vi "Diagnostics.Main.CmdResp.Engine.vi"(8 "error in (no error)":errorcluster, 11 "State Variables":T1={"Comm"=refnum, "Parameters"={"Properties"={"Name"="", "CAN"={"Interface"="", "Baud Rate"=0, "Diagnostic Protocol"=enum."GMLAN", "Transport Protocol"=enum."ISO TP - Normal Mode", "Transmit ID"=0, "Receive ID"=0, "Transmit Extension"=2, "Receive Extension"=1, "Receive UUDT ID"=0, "Enable Stream"=TRUE, "VW TP Channel ID"=0, "Fill Frame"=FALSE, "Fill Byte"=255, "Termination"=FALSE, "LIN Cluster"="ADCS_LIN_database", "NAD"=1, "IO Mode"=0, "Max DLC"=8, "FD Baud Rate"=0, "Security"={"Type"=enum."None", "Source DLL Path"=path "", "Target DLL Path"=path "", "Security Level"=0, "Master Key"=""}, "Timeout"=0}, "986x"={"Enable"=FALSE, "RIO Device"="", "Bitfile"=path ""}, "Reads"=[], "Frames Lookup"=variant(enum16{"GMLAN", "KWP-2000", "UDS"} enum."GMLAN"), "Writes"=[], "DPIDs"=[], "DPID Lookup"=variant(u32 0), "DTC"={"Descriptor"={"DTC Byte Length"=2, "Status Byte Length"=1, "Add Data Byte Length"=1, "Byte Order"=enum."Motorola"}, "Value.Code"=[], "Value.String"=[], "Value.J2012String"=[], "Status.Code"=[], "Status.String"=[]}, "Created DTCs"=0, "Polls"=[], "Service Channels Status Lookup"=variant, "Trigger Lookup"=variant}}, "ADCS Connection"={"Diag CAN Handle"=0, "Transport Protocol"=enum."ISO TP - Normal Mode", "Receive Address Extension"=0, "Transmit Address Extension"=0, "Receive CAN Id"=0, "Transmit CAN Id"=0, "Log Frames ?"=FALSE, "My TP Address"=0, "Other TP Address"=0, "T1"=0, "T2"=0, "T3"=0, "T4"=0, "Tx SN"=0, "Block Size"=0, "Rx SN"=0, "VW TP Initialized?"=FALSE, "Tx block no"=0, "baud rate"=0, "Interface"="", "Channel Diag CAN Handle"=0, "UDP Connection ID"=refnum, "TCP Connection ID"=refnum, "Target IP Addr"=0, "Source Address"=0, "Target Address"=0, "Send Header NACK?"=FALSE, "DLL Handle"=0, "NAD"=0, "Time Stamp read first"=0.0, "Time Stamp read last"=0.0, "Time Stamp write first"=0.0, "Time Stamp write last"=0.0, "Time Stamp write"=0.0, "Time Stamp read"=0.0, " I/O Mode"=0, "FD Baudrate"=0, "TX_DL"=8, "RX_DL"=8, "DoIP Protocol Version"=1, " Selected I/O Mode"=0, "TesterPresent Counter"=0, "TesterPresent Limit"=0, "TesterPresent Tick[ms]"=10, "TesterPresent RequireResponse?"=FALSE, "TesterPresent Stored Ref?"=FALSE, "TesterPresent Message"=[], "TesterPresent Task Handle"=0, "TesterPresent Semaphore"=refnum, "Response Plausibility Check"=1, "Default Version?"=TRUE, "Diagostic Globals"={"Timeout FC (Bs)"=250, "Timeout CF (Cr)"=250, "Timeout Diag Command"=1000, "Receive Block Size (BS)"=0, "Wait Time CF (STmin)"=5, "Max Waits (N_WFTmax)"=10, "Waits to Send (N_WAIT)"=0, "Time between Waits (TW)"=25, "Fill CAN Frames?"=TRUE, "Fill Byte"=255, "Invalid Response as Error?"=FALSE, "Max RspPending Count"=5, "VWTP Command Timeout"=50, "Transport Protocol"=enum."Diagnostics on IP", "Diag CAN Handle"=0, "DLL Handle"=0, "Timeout RspPending"=1000}, "Session-based Properties?"=FALSE}, "XNET References"={"Database"="", "GMLAN DPID Session"="", "Cluster"=""}, "XNETEngine (GMLAN)"=refnum, "Process"=refnum, "Reads"=refnum, "Writes"=refnum, "Cmds"=refnum, "DTCs"=refnum, "DTC Count"=refnum, "Status"=refnum, "Triggers"=refnum, "CANConnected"=refnum, "LocalStop"=refnum, "LocalCommStatus"=refnum, "Service Channels Status"=refnum, "Settings"=refnum} {"ADCS Connection"."Diagostic Globals"."Fill Byte" format="%x"; "ADCS Connection"."TesterPresent Message" format="%.0x"; "ADCS Connection"."Selected I/O Mode" items=["CAN", "CAN FD", "CAN FD+BRS", "ECU Determined"]; "ADCS Connection"."DoIP Protocol Version" items=["2010"=1, "2012"=2]; "ADCS Connection"."RX_DL" items=["8"=8, "12"=12, "16"=16, "20"=20, "24"=24, "32"=32, "48"=48, "64"=64]; "ADCS Connection"."TX_DL" items=["8"=8, "12"=12, "16"=16, "20"=20, "24"=24, "32"=32, "48"=48, "64"=64]; "ADCS Connection"."I/O Mode" items=["CAN", "CAN FD", "CAN FD+BRS", "Not yet determined"]; "Parameters"."Properties"."Writes"."Signals"."Byte Order" items=["Little Endian", "Big Endian"]; "Parameters"."Properties"."Writes"."Signals"."Data Type" items=["Signed", "Unsigned", "IEEE Float"]; "Parameters"."Properties"."CAN"."IO Mode" items=["CAN 2.0", "CAN FD", "CAN FD+BRS"]; "Parameters"."Properties"."CAN"."Fill Byte" format="%.0x"; "Parameters"."Properties"."CAN"."VW TP Channel ID" format="%.0x"; "Parameters"."Properties"."CAN"."Receive UUDT ID" format="%.0x"; "Parameters"."Properties"."CAN"."Receive Extension" format="%.0x"; "Parameters"."Properties"."CAN"."Transmit Extension" format="%.0x"; "Parameters"."Properties"."CAN"."Receive ID" format="%.0x"; "Parameters"."Properties"."CAN"."Transmit ID" format="%.0x"; "Parameters"."Properties"."Reads"."Signals"."Byte Order" items=["Little Endian", "Big Endian"]; "Parameters"."Properties"."Reads"."Signals"."Data Type" items=["Signed", "Unsigned", "IEEE Float"]}) -> (0 "error out":errorcluster)   [LabVIEW 2019, in "Diagnostics Addon Engine.lvlib"]
doc: "Async loop that handles the UDS commands sent either by the channel engine or the TCP engine"
uses:
  Diagnostics Addon Engine.lvlib
  <vilib>/NI VeriStand/Custom Device Tools/Custom Device Utility Library/Custom Device Utility Library.lvlib
  Shared/Types/DTC.Info.ctl
  Shared/Diagnostics Addon Shared.lvlib
  <vilib>/NI/AMC/AMC.lvlib
  GMLAN/GMLAN.lvlib
  GMLAN/_SubVIs/InitiateDiagnosticOperation_Parameter.ctl
  GMLAN/_SubVIs/InitiateDiagnosticOperation_SubFunctions.ctl
  GMLAN/_SubVIs/ReadDataByPacketIdentifier_SubFunctions.ctl
  <vilib>/Automotive Diagnostic Command Set/Diagnostic Transport.llb/Property ID.ctl
  <vilib>/addons/Automotive Diagnostic Command Set/NI_Automotive Diagnostic Command Set.lvlib
  Types/Frame.Data.ctl
  Shared/Types/Command.ReadDTCbyDTCNumber.ctl
  GMLAN/_SubVIs/ReadFailureRecordData_readFailureRecordParameters_failureRecordIdentifier.ctl
  Shared/Types/Command.IO.ctl
  Shared/Types/Type.ctl
  GMLAN/_SubVIs/TesterPresent_Parameter.ctl
  Shared/Types/Command.Communication.ctl
  Shared/Types/Command.Memory.ctl
  Shared/Types/Command.PassThru.Channel.ctl
  Shared/Types/Command.ReadDTC.ctl
  GMLAN/_SubVIs/DisableNormalCommunication_Parameter.ctl
  <vilib>/NI/NIVS Inline Async API/_VS Inline Async API/Process/Process.lvclass
  <vilib>/NI/NIVS Inline Async API/_Data Access Engine/Data Access Engine/Data Access Engine.lvclass
  <vilib>/NI/NIVS Inline Async API/_Data Access Engine/Data Access Engine/Methods/Write.Data.vi
  <vilib>/NI/NIVS Addon Network Comm/Engine/VeriStand Comm.lvclass
  Shared/Types/DTC.Descriptor.Override.ctl
  Shared/Types/Command.ClearDTC.ctl
  Shared/Types/Command.ControlDTC.ctl
  <vilib>/NI/NIVS Inline Async API/_Data Access Engine/Data Access Engine/Methods/Write.Data.Commit.vi
  Types/Polling.States.ctl
  Shared/Types/Signal.ctl
  Shared/Types/DPID.Rate.ctl
  Shared/Types/DPID.ctl
  Shared/Types/Protocol.ctl
  Shared/Types/CAN.Interface.ctl
  Shared/Types/CAN.ctl
  Shared/Types/SysDef.Compile.Properties.ctl
  Types/XNET.Refs.ctl
  Types/Diagnostics.State.ctl
  <vilib>/NI/Tools/Keyed Array/KeyedArray.ctl
  <vilib>/NI/Tools/Keyed Array/Tools_KeyedArray.lvlib
  <vilib>/NI/AMC/Message.ctl
  <vilib>/NI/AMC/Message Queue.ctl
  Shared/Types/Transport.ctl
  <vilib>/Automotive Diagnostic Command Set/Diagnostic Transport.llb/Transport Protocol Selector.ctl
  <vilib>/Automotive Diagnostic Command Set/Diagnostic Transport.llb/Diag Reference.ctl
  Shared/Types/Security.ctl
  Shared/Types/Frame.Compile.ctl
  Shared/Types/DTC.Settings.ctl
  Shared/Types/986x.ctl
  <vilib>/NI/NIVS Inline Async API/_Data Access Engine/Access Type Classes/ReadWrite/ReadWrite.lvclass
  Shared/Types/SysDef.Compile.ctl
  <vilib>/NI/NIVS Inline Async API/_Data Access Engine/Access Type Classes/Write/Write.lvclass
  <vilib>/NI/NIVS Inline Async API/_Data Access Engine/Data Access Engine/Types/Write.DVR.ctl
  <vilib>/NI/NIVS Inline Async API/_Data Access Engine/Access Type Classes/Read/Read.lvclass
  <vilib>/NI/NIVS Inline Async API/_Data Access Engine/Data Access Engine/Types/Read.DVR.ctl
  <vilib>/NI/NIVS Inline Async API/_Data Access Engine/Data Access Engine/Types/ReadWrite.DVR.ctl
  Shared/Types/DTC.Descriptor.ctl
  <vilib>/Automotive Diagnostic Command Set/Diagnostic Transport.llb/DoIP Protocol Version.ctl
  <vilib>/Automotive Diagnostic Command Set/Diagnostic Transport.llb/Diag Globals.ctl
  Shared/Types/Security.Type.ctl
  Shared/Types/Poll.Compiled.ctl
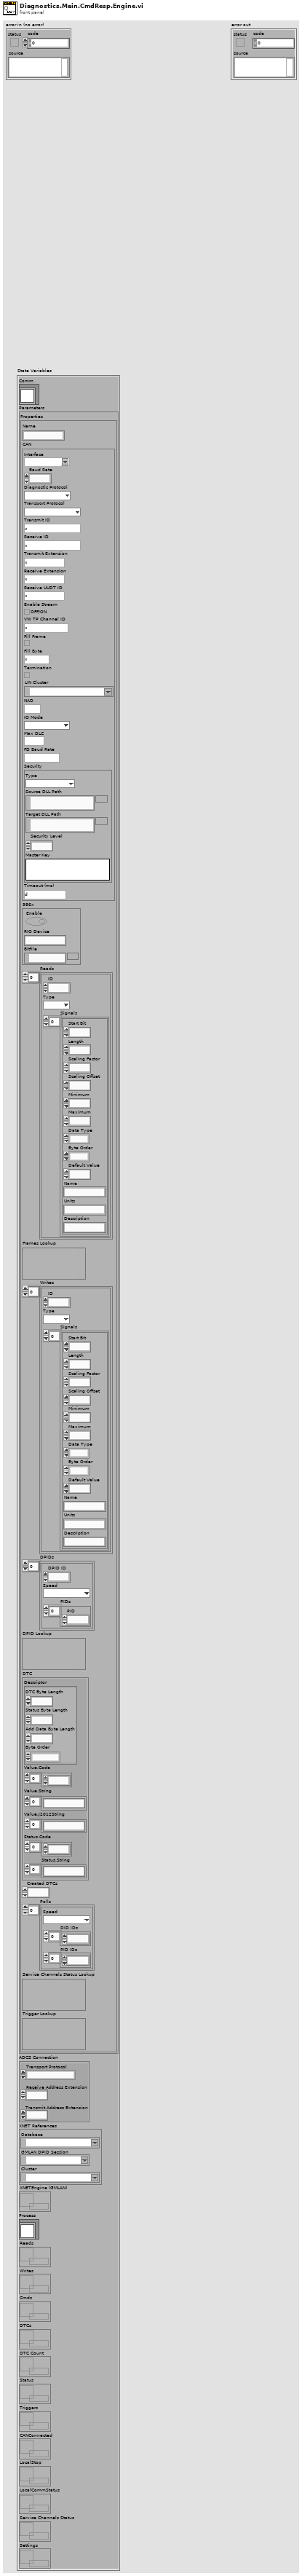
[diagram p1: front panel]
types:
  T1 = typedef "Diagnostics Addon Engine.lvlib/Diagnostics.State.ctl" = cluster{"Comm":refnum<class "VeriStand Comm.lvclass">, "Parameters":T2, "ADCS Connection":T19, "XNET References":T24, "XNETEngine (GMLAN)":T25, "Process":refnum<class "Process.lvclass">, "Reads":T26, "Writes":T27, "Cmds":T28, "DTCs":T26, "DTC Count":T26, "Status":T26, "Triggers":T28, "CANConnected":T26, "LocalStop":refnum<data-value>, "LocalCommStatus":refnum<data-value>, "Service Channels Status":T26, "Settings":T27}
  T2 = typedef "Diagnostics Addon Shared.lvlib/SysDef.Compile.ctl" = cluster{"Properties":T3}
  T3 = typedef "Diagnostics Addon Shared.lvlib/SysDef.Compile.Properties.ctl" = cluster{"Name":string, "CAN":T4, "986x":T10, "Reads":T11[], "Frames Lookup":variant, "Writes":T11[], "DPIDs":T14[], "DPID Lookup":variant, "DTC":T16, "Created DTCs":u32, "Polls":T18[], "Service Channels Status Lookup":variant, "Trigger Lookup":variant}
  T4 = typedef "Diagnostics Addon Shared.lvlib/CAN.ctl" = cluster{"Interface":T5, "Baud Rate":u64, "Diagnostic Protocol":T6, "Transport Protocol":T7, "Transmit ID":u32, "Receive ID":u32, "Transmit Extension":u8, "Receive Extension":u8, "Receive UUDT ID":u32, "Enable Stream":bool, "VW TP Channel ID":u32, "Fill Frame":bool, "Fill Byte":u8, "Termination":bool, "LIN Cluster":refnum<k21>, "NAD":u8, "IO Mode":u32, "Max DLC":u16, "FD Baud Rate":u64, "Security":T8, "Timeout":u32}
  T5 = typedef "Diagnostics Addon Shared.lvlib/CAN.Interface.ctl" = string
  T6 = typedef "Diagnostics Addon Shared.lvlib/Protocol.ctl" = enum16{"GMLAN", "KWP-2000", "UDS", "User-Defined"}
  T7 = typedef "Diagnostics Addon Shared.lvlib/Transport.ctl" = enum16{"ISO TP - Normal Mode", "ISO TP - Mixed Mode", "VW TP 2.0", "Diagnostics on IP", "ISO TP LIN"}
  T8 = typedef "Diagnostics Addon Shared.lvlib/Security.ctl" = cluster{"Type":T9, "Source DLL Path":path, "Target DLL Path":path, "Security Level":u8, "Master Key":string}
  T9 = typedef "Diagnostics Addon Shared.lvlib/Security.Type.ctl" = enum16{"None", "DLL", "MasterKey"}
  T10 = typedef "Diagnostics Addon Shared.lvlib/986x.ctl" = cluster{"Enable":bool, "RIO Device":string, "Bitfile":path}
  T11 = typedef "Diagnostics Addon Shared.lvlib/Frame.Compile.ctl" = cluster{"ID":u32, "Type":T12, "Signals":T13[]}
  T12 = typedef "Diagnostics Addon Shared.lvlib/Type.ctl" = enum16{"DID", "CDID", "PID", "CPID", "Read Memory", "Write Memory", "DTC Control", "IO Control", "Routine Start", "Routine Request", "Routine Stop", "User Defined", "Tester Present", "Clear DTCs", "Read DTCs", "Start DTCs", "DTC Change Count", "Unlock ECU", "Reset ECU", "Diagnostic Session Control", "Normal Communication Control", "Configure and Start DPIDs", "Stop DPIDs"}
  T13 = typedef "Diagnostics Addon Shared.lvlib/Signal.ctl" = cluster{"Start Bit":u32, "Length":u32, "Scaling Factor":dbl, "Scaling Offset":dbl, "Minimum":dbl, "Maximum":dbl, "Data Type":u32, "Byte Order":u32, "Default Value":dbl, "Name":string, "Units":string, "Description":string}
  T14 = typedef "Diagnostics Addon Shared.lvlib/DPID.ctl" = cluster{"DPID ID":u8, "Speed":T15, "PIDs":u16[]}
  T15 = typedef "Diagnostics Addon Shared.lvlib/DPID.Rate.ctl" = enum16{"Slow", "Medium", "Fast"}
  T16 = typedef "Diagnostics Addon Shared.lvlib/DTC.Settings.ctl" = cluster{"Descriptor":T17, "Value.Code":dbl[], "Value.String":string[], "Value.J2012String":string[], "Status.Code":dbl[], "Status.String":string[]}
  T17 = typedef "Diagnostics Addon Shared.lvlib/DTC.Descriptor.ctl" = cluster{"DTC Byte Length":i32, "Status Byte Length":i32, "Add Data Byte Length":i32, "Byte Order":enum16{"Motorola", "Intel"}}
  T18 = typedef "Diagnostics Addon Shared.lvlib/Poll.Compiled.ctl" = cluster{"Speed":T15, "DID IDs":u32[], "PID IDs":u32[]}
  T19 = typedef "NI_Automotive Diagnostic Command Set.lvlib/Diag Reference.ctl" = cluster{"Diag CAN Handle":u32, "Transport Protocol":T20, "Receive Address Extension":u8, "Transmit Address Extension":u8, "Receive CAN Id":u32, "Transmit CAN Id":u32, "Log Frames ?":bool, "My TP Address":u8, "Other TP Address":u8, "T1":u16, "T2":u16, "T3":u16, "T4":u16, "Tx SN":u8, "Block Size":u8, "Rx SN":u8, "VW TP Initialized?":bool, "Tx block no":u8, "baud rate":u64, "Interface":string, "Channel Diag CAN Handle":u32, "UDP Connection ID":refnum<k16>, "TCP Connection ID":refnum<k5>, "Target IP Addr":u32, "Source Address":u16, "Target Address":u16, "Send Header NACK?":bool, "DLL Handle":u32, "NAD":u8, "Time Stamp read first":dbl, "Time Stamp read last":dbl, "Time Stamp write first":dbl, "Time Stamp write last":dbl, "Time Stamp write":dbl, "Time Stamp read":dbl, " I/O Mode":u32, "FD Baudrate":u64, "TX_DL":u16, "RX_DL":u16, "DoIP Protocol Version":T21, " Selected I/O Mode":u32, "TesterPresent Counter":u32, "TesterPresent Limit":u32, "TesterPresent Tick[ms]":i32, "TesterPresent RequireResponse?":bool, "TesterPresent Stored Ref?":bool, "TesterPresent Message":u8[], "TesterPresent Task Handle":i32, "TesterPresent Semaphore":T22, "Response Plausibility Check":u32, "Default Version?":bool, "Diagostic Globals":T23, "Session-based Properties?":bool}
  T20 = typedef "NI_Automotive Diagnostic Command Set.lvlib/Transport Protocol Selector.ctl" = enum16{"ISO TP - Normal Mode", "ISO TP - Mixed Mode", "VW TP 2.0", "Diagnostics on IP", "ISO TP LIN"}
  T21 = typedef "NI_Automotive Diagnostic Command Set.lvlib/DoIP Protocol Version.ctl" = u8
  T22 = typedef "Semaphore RefNum" = refnum<k1>
  T23 = typedef "NI_Automotive Diagnostic Command Set.lvlib/Diag Globals.ctl" = cluster{"Timeout FC (Bs)":u32, "Timeout CF (Cr)":u32, "Timeout Diag Command":u32, "Receive Block Size (BS)":u8, "Wait Time CF (STmin)":u8, "Max Waits (N_WFTmax)":u8, "Waits to Send (N_WAIT)":i32, "Time between Waits (TW)":u32, "Fill CAN Frames?":bool, "Fill Byte":u32, "Invalid Response as Error?":bool, "Max RspPending Count":u32, "VWTP Command Timeout":u32, "Transport Protocol":T20, "Diag CAN Handle":u32, "DLL Handle":u32, "Timeout RspPending":u32}
  T24 = typedef "Diagnostics Addon Engine.lvlib/XNET.Refs.ctl" = cluster{"Database":refnum<k21>, "GMLAN DPID Session":refnum<k21>, "Cluster":refnum<k21>}
  T25 = typedef "AMC.lvlib/Message Queue.ctl" = refnum<queue>
  T26 = typedef "Data Access Engine.lvlib/Data Access Engine.lvclass/Write.DVR.ctl" = refnum<data-value>
  T27 = typedef "Data Access Engine.lvlib/Data Access Engine.lvclass/Read.DVR.ctl" = refnum<data-value>
  T28 = typedef "Data Access Engine.lvlib/Data Access Engine.lvclass/ReadWrite.DVR.ctl" = refnum<data-value>
  T29 = typedef "Diagnostics Addon Engine.lvlib/Polling.States.ctl" = cluster{"Enabled":bool[], "Last Generation":u32[], "Queued":bool[]}
  T30 = typedef "Diagnostics Addon Shared.lvlib/DTC.Info.ctl" = cluster{"Timestamp":dbl, "DTC":dbl, "Status":dbl, "Add Data":dbl}
  T31 = cluster{"Active DTCs":T30[], "status mask":u8, "PID IDs":u32[], "DID IDs":u32[], "Memory IDs":u32[], "TesterPresentEnabled?":bool, "Polling":T29}
  T32 = typedef "NI_Automotive Diagnostic Command Set.lvlib/Property ID.ctl" = enum16{"Timeout Diag Command", "Timeout FC (Bs)", "Timeout CF (Cr)", "Receive Block Size (BS)", "Wait Time CF (STmin)", "Max Wait Frames (N_WFTmax)", "Wait Frames to Send (N_WAIT)", "Time between Waits (T_W)", "Fill CAN Frames", "Fill Byte", "Invalid Response as Error", "Max RspPending Count", "VWTP Command Timeout", "STmin", "P2min", "Termination", "Timeout RspPending", "LIN Sleep", "Actual CAN IO Mode", "Response Plausibility Check", "Session-based Properties"}
  T33 = typedef "GMLAN.lvlib/ReadFailureRecordData_readFailureRecordParameters_failureRecordIdentifier.ctl" = cluster{"failureRecordNumber":u8, "DTC ID":u16, "DTCFailureType":u8}
  T34 = enum16{"open", "replace", "create", "open or create", "replace or create", "replace or create with confirmation"}
  T35 = typedef "Diagnostics Addon Shared.lvlib/Command.ReadDTCbyDTCNumber.ctl" = cluster{"DTC":u16, "FailTypeByte":u8}
  T36 = typedef "Diagnostics Addon Engine.lvlib/Frame.Data.ctl" = cluster{"ID":u32, "Raw Frame":u8[], "error out":errorcluster}
  T37 = typedef "GMLAN.lvlib/ReadDataByPacketIdentifier_SubFunctions.ctl" = enum8{"stopSending", "sendOneResponse", "scheduleAtSlowRate", "scheduleAtMediumRate", "scheduleAtFastRate"}
  T38 = typedef "GMLAN.lvlib/TesterPresent_Parameter.ctl" = enum8{"SpecificECU", "EntireNetwork"}
  T39 = typedef "GMLAN.lvlib/InitiateDiagnosticOperation_Parameter.ctl" = enum8{"SpecificECU", "EntireNetwork"}
  T40 = typedef "Diagnostics Addon Shared.lvlib/Command.Communication.ctl" = cluster{"Type":u8, "CommType":u8}
  T41 = typedef "GMLAN.lvlib/DisableNormalCommunication_Parameter.ctl" = enum8{"SpecificECU", "EntireNetwork"}
  T42 = typedef "Diagnostics Addon Shared.lvlib/Command.ReadDTC.ctl" = cluster{"Extension":u32, "Mask":u32, "Mode":u32, "Byte Lengths":T43}
  T43 = typedef "Diagnostics Addon Shared.lvlib/DTC.Descriptor.Override.ctl" = cluster{"Override":bool, "DTC":u32, "Status":u32, "Failure":u32}
  T44 = typedef "Diagnostics Addon Shared.lvlib/Command.ClearDTC.ctl" = cluster{"Group of DTC":u32, "Byte Lengths":T43}
  T45 = typedef "Diagnostics Addon Shared.lvlib/Command.PassThru.Channel.ctl" = cluster{"Service":u64, "Service Length":u8, "Data Length":u32, "Response Required":bool}
  T46 = cluster{"resp":u8[], "error code":u8, "error out":errorcluster}
  T47 = typedef "Diagnostics Addon Shared.lvlib/Command.ControlDTC.ctl" = cluster{"Group/Type":u32, "Byte Lengths (KWP only)":T43}
  T48 = typedef "Diagnostics Addon Shared.lvlib/Command.Memory.ctl" = cluster{"Address":u64, "Service Type":u32, "Address Length":u8, "Size Length":u8}
  T49 = typedef "Diagnostics Addon Shared.lvlib/Command.IO.ctl" = cluster{"ID":u16, "Mode":u8}
  T50 = typedef "NI VeriStand Addon Network Comm.lvlib/VeriStand Comm.lvclass/Response Information.ctl" = cluster{"response name":string, "responseQ":string}
  T51 = cluster{"Boolean array[0]":bool, "Boolean array[1]":bool, "Boolean array[2]":bool, "Boolean array[3]":bool, "Boolean array[4]":bool, "Boolean array[5]":bool, "Boolean array[6]":bool, "Boolean array[7]":bool}
  T52 = typedef "Diagnostics Addon Engine.lvlib/DPIDs.IDs.Sorted.ctl" = cluster{"Slow":u8[], "Medium":u8[], "Fast":u8[]}
  T53 = typedef "GMLAN.lvlib/InitiateDiagnosticOperation_SubFunctions.ctl" = u8
  T54 = typedef "Diagnostic Trouble Code.ctl" = cluster{"DTC":u32, "Status":u32, "Add Data":u32}
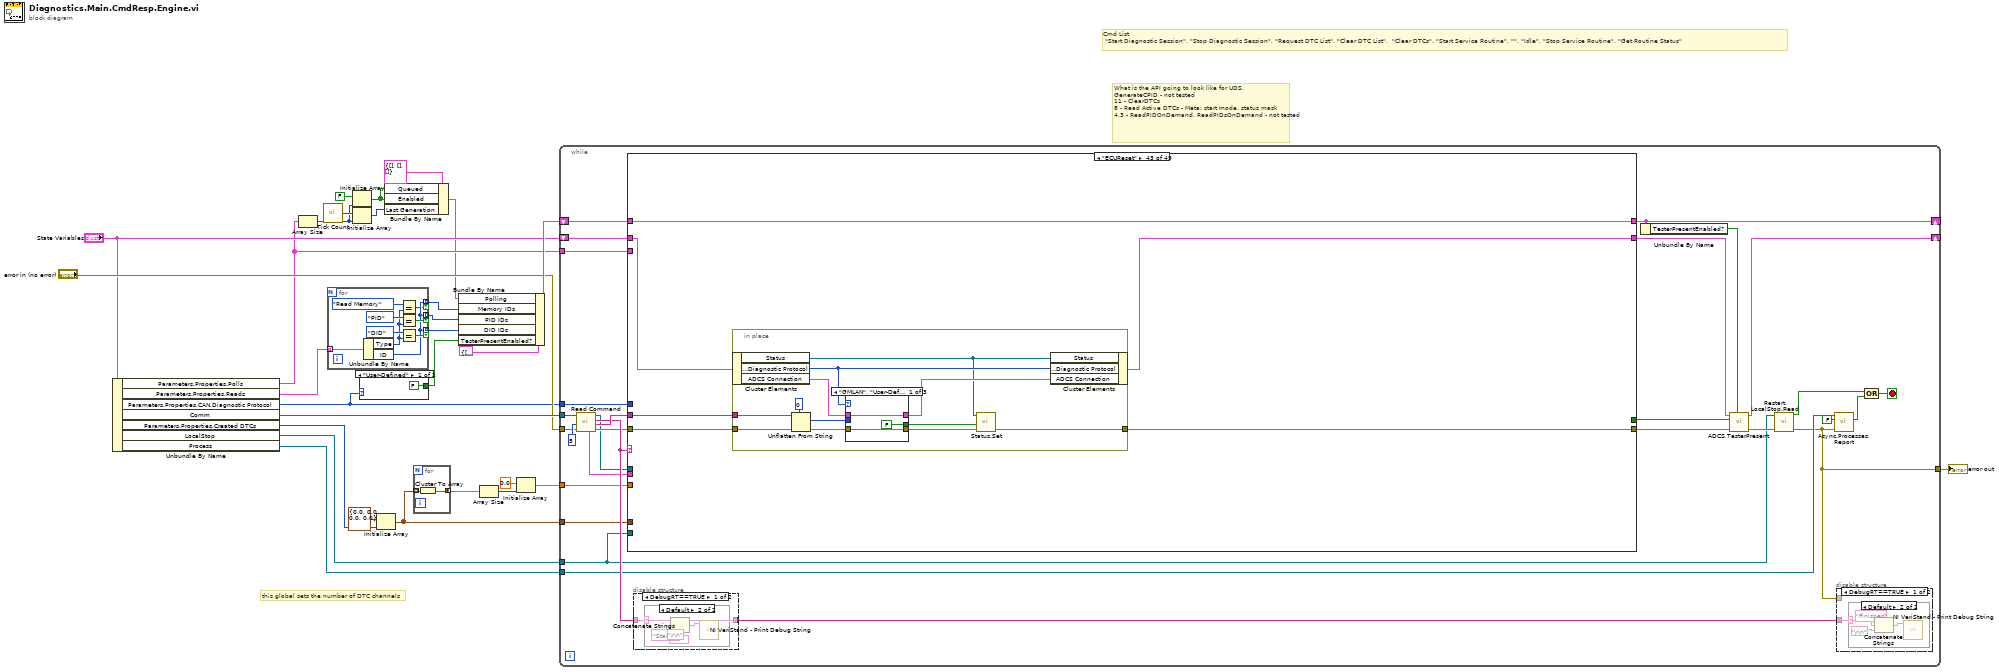
[diagram p0: block diagram]
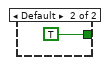
[diagram p2: hidden frame]
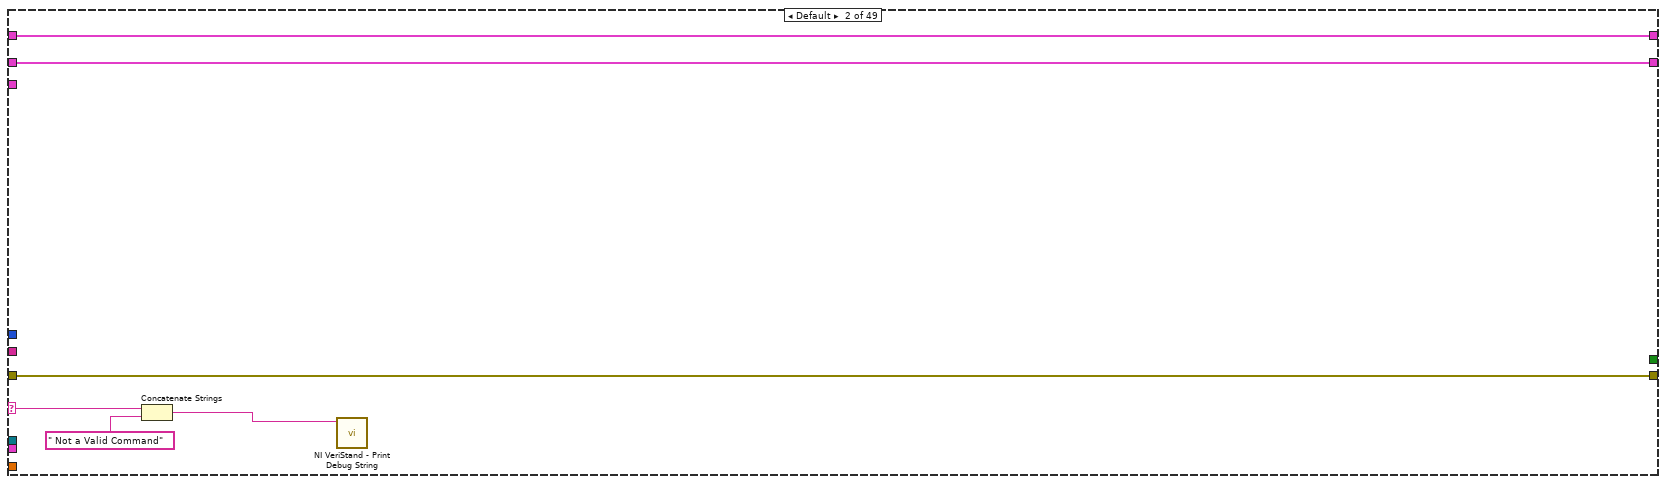
[diagram p8: hidden frame]
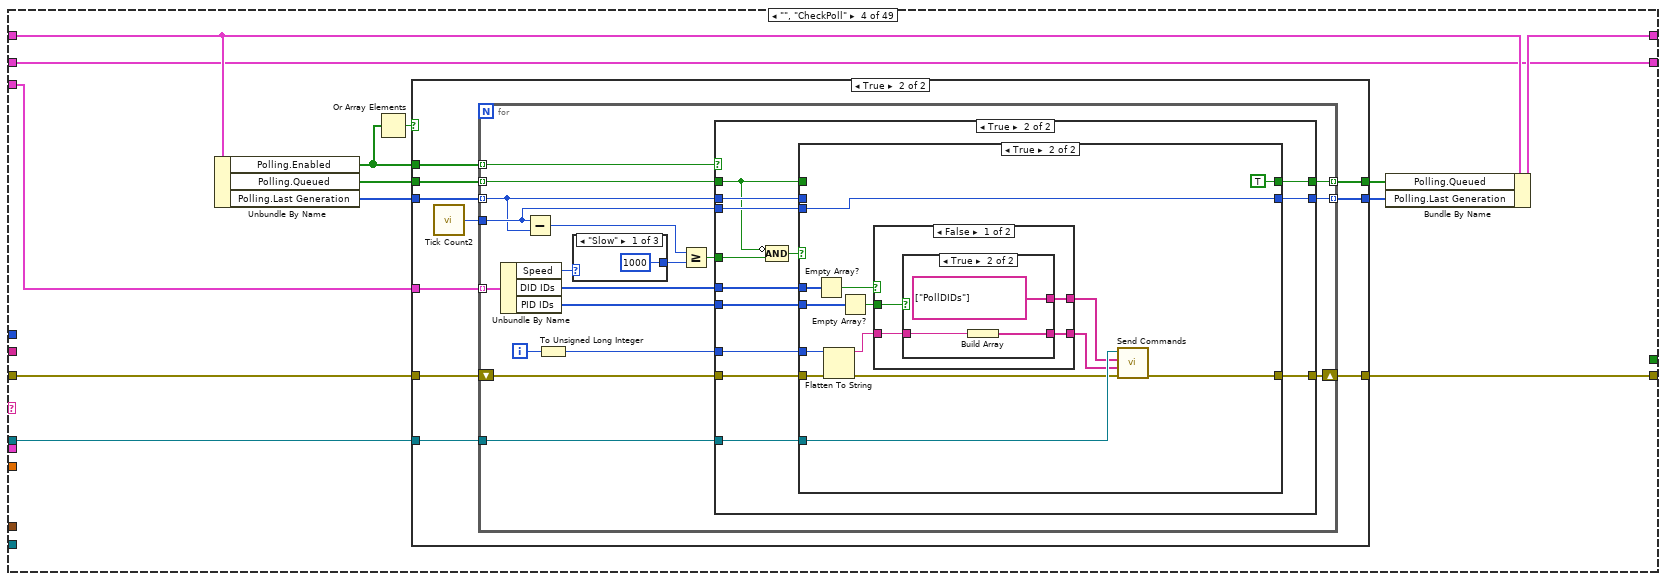
[diagram p10: hidden frame]
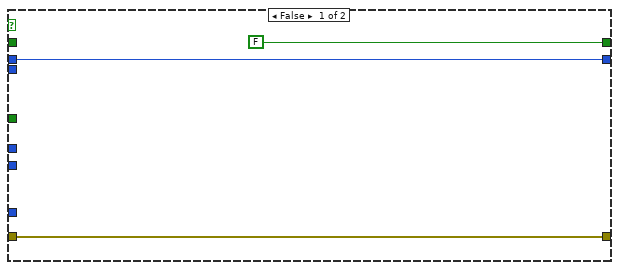
[diagram p12: hidden frame]
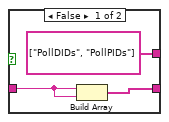
[diagram p14: hidden frame]
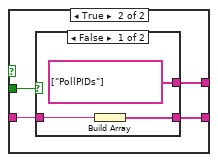
[diagram p15: hidden frame]
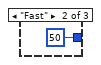
[diagram p17: hidden frame]
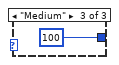
[diagram p18: hidden frame]
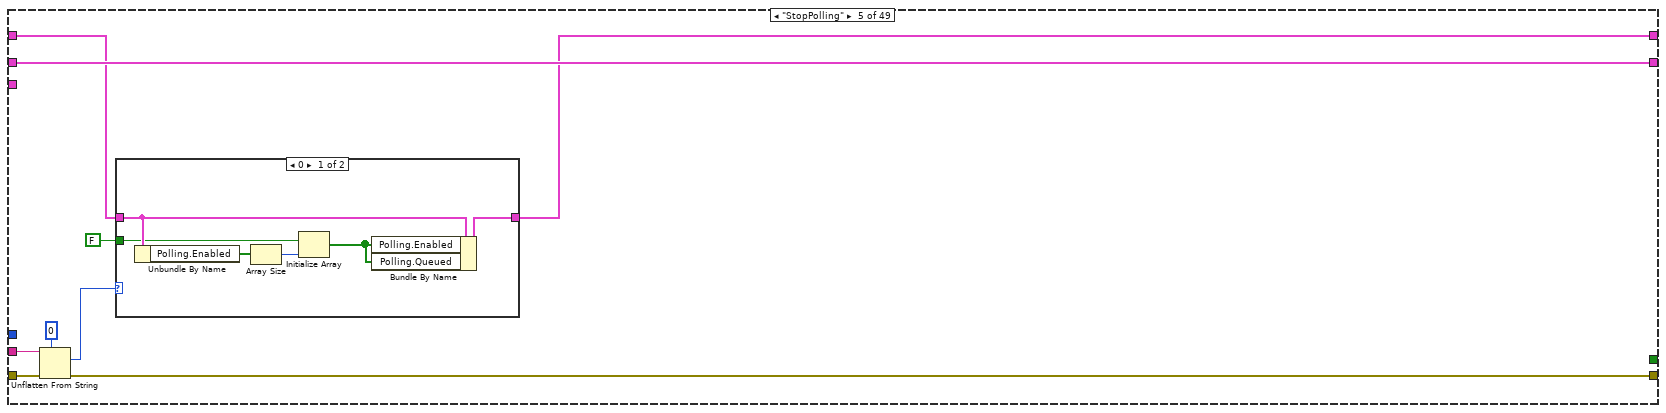
[diagram p19: hidden frame]
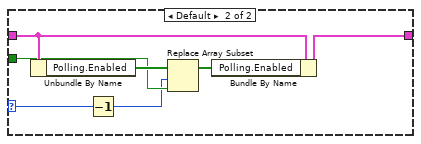
[diagram p20: hidden frame]
diagram:
  # "this global sets the number of DTC channels"
  # "What is the API going to look like for UDS.\nGenerateCPID - not tested\n11 - ClearDTCs\n8 - Read Active DTCs - Meta: start mode, status mask \n4,3 - ReadPIDOnDemand, ReadPIDsOnDemand - not tested"
  # "Cmd List\n \"Start Diagnostic Session\", \"Stop Diagnostic Session\", \"Request DTC List\", \"Clear DTC List\",  \"Clear DTCs\", \"Start Service Routine\", \"\", \"Idle\", \"Stop Service Routine\", \"Get Routine Status\""
  n1 = Unbundle By Name("State Variables") -> ("Parameters.Properties.Polls"=w5:T18[], "Parameters.Properties.Reads"=w26:T11[], "Parameters.Properties.CAN.Diagnostic Protocol"=w2:T6, "Comm"=w28:refnum<class "VeriStand Comm.lvclass">, "Parameters.Properties.Created DTCs"=w19:u32, "LocalStop"=w12:refnum<data-value>, "Process"=w18:refnum<class "Process.lvclass">)
  n2 = Array Size(array=w5) -> (size(s)=w6:i32)
  n3 = call "Tick Count"() -> ("Tick Count(mSec)"=w9:u32)
  n4 = for {
    tunnel: w26 -> [w38] mode=indexing
    tunnel: [w31] -> w22 mode=indexing if=w35
    tunnel: [w31] -> w23 mode=indexing if=w34
    tunnel: [w31] -> w21 mode=indexing if=w30
    n5 = Unbundle By Name(w38) -> ("Type"=w33:T12, "ID"=w31:u32)
    n6 = Equal?(x=Type."Read Memory", y=w33) -> (x = y?=w30:bool)
    n7 = Equal?(x=Type."PID", y=w33) -> (x = y?=w34:bool)
    n8 = Equal?(x=Type."DID", y=w33) -> (x = y?=w35:bool)
  }
  n9 = Initialize Array(FALSE, w6) -> (w1:bool[])
  n10 = Initialize Array(w9, w6) -> (w8:u32[])
  n11 = case shown="\"User-Defined\"" w2 {
    tunnel: [FALSE ("TesterPresentEnabled?") TRUE ("TesterPresentEnabled?")] -> w20
    frame "User-Defined" {
    }
    frame Default {
    }
  }
  n12 = Initialize Array(T30 {"Timestamp"=0.0, "DTC"=0.0, "Status"=0.0, "Add Data"=0.0} ("Diagnostic Trouble Code"), w19) -> (w17:T30[])
  n13 = Bundle By Name(cluster=T29 {"Enabled"=[], "Last Generation"=[], "Queued"=[]}, "Queued"=w1, "Enabled"=w1, "Last Generation"=w8) -> (w3:T29)
  n14 = for {
    tunnel: w17 -> [w42] mode=indexing
    tunnel: [w41] -> w16 mode=concatenating
    # "Put 10 newest DTCs in VS"
    n15 = Cluster To Array(cluster=w42) -> (array=w41:dbl[])
  }
  n16 = Bundle By Name(cluster=T31 {"Active DTCs"=[], "status mask"=0, "PID IDs"=[], "DID IDs"=[], "Memory IDs"=[], "TesterPresentEnabled?"=FALSE, "Polling"={"Enabled"=[], "Last Generation"=[], "Queued"=[]}}, "Polling"=w3, "Memory IDs"=w21, "PID IDs"=w23, "DID IDs"=w22, "TesterPresentEnabled?"=w20) -> (w24:T31)
  n17 = Array Size(array=w16) -> (size(s)=w15:i32)
  n18 = Initialize Array(0.0 ("element"), w15) -> (w13:dbl[])
  n19 = while {
    tunnel: w28 -> [w71]
    tunnel: "error in (no error)" -> [w69]
    tunnel: [w49] -> w29
    tunnel: w18 -> [w54]
    shift-right: [w56] -> _
    shift-left: w24 -> [w67]
    tunnel: w17 -> [w64]
    shift-right: [w61] -> _
    shift-left: "State Variables" -> [w63]
    tunnel: w13 -> [w52]
    tunnel: w12 -> [w45]
    tunnel: w5 -> [w44]
    tunnel: w2 -> [w43]
    stop <- w46 stop-if-true
    n20 = call <vilib>:"Read Command.vi"("error in (no error)"=w69, "timeout (100 ms)"=5 ("timeout (1ms)"), "VeriStand Comm in"=w71) -> ("error out"=w60:errorcluster, "message value"=w68:string, "message name"=w66:string, "VeriStand Comm out"=w51:refnum<class "VeriStand Comm.lvclass">, "ResponseInfo"=w65:T50)  [unwired: 3 in, 1 out]
    n21 = case shown="\"ECUReset\"" w66 {
      selector: w66 -> [_ w87 _ _ _ _ _ w246 _ _ _ _ _ _ _ _ _ _ _ _ _ _ _ _ _ _ _ _ _ _ _ w1350 _ _ w1596 _ w1702 _ _ _ _ _ _ _ _ _ _ _ _]
      tunnel: w60 -> [w85 w91 w94 w106 w193 w215 w238 w248 w302 w347 w400 w413 w457 w493 w566 w664 w757 w816 w873 w920 w927 w937 w942 w948 w990 w1000 w1038 w1073 w1118 w1153 w1181 w1347 w1450 w1525 w1595 w1652 w1700 w1736 w1783 w1789 w1832 w1837 w1885 w1918 w1992 w2061 w2146 w2194 w2240]
      tunnel: w68 -> [_ _ _ _ w195 w217 _ w245 w300 w348 w397 w414 _ _ w560 _ w756 _ w872 _ _ _ _ w944 _ w998 _ w1070 _ _ w1180 w1348 w1446 _ w1594 w1651 w1701 w1735 _ w1790 _ w1835 w1883 w1916 w1990 w2060 w2142 w2193 w2239]
      tunnel: [w85 w91 w94 w105 w194 w216 w238 w247 w301 w346 w399 w412 w456 w492 w565 w663 w755 w815 w871 w920 w926 w937 w942 w947 w989 w999 w1039 w1074 w1119 w1152 w1183 w1349 w1449 w1524 w1593 w1650 w1703 w1732 w1783 w1791 w1832 w1836 w1884 w1917 w1991 w2059 w2145 w2192 w2237] -> w58
      tunnel: [w84 w90 w93 w101 w198 w220 w240 w241 w296 w349 w398 w415 w458 w496 w561 w660 w752 w817 w874 w922 w923 w935 w939 w950 w991 w1001 w1040 w1075 w1120 w1154 w1176 w1341 w1444 w1521 w1590 w1653 w1705 w1737 w1785 w1793 w1834 w1840 w1886 w1919 w1993 w2062 w2147 w2195 w2242] -> w56
      tunnel: w67 -> [w84 w90 w93 w100 w197 w219 w240 w244 w297 w349 w396 w415 w458 w496 w562 w660 w752 w817 w874 w922 w924 w936 w940 w950 w991 w1001 w1040 w1075 w1120 w1154 w1177 w1344 w1443 w1521 w1590 w1653 w1705 w1737 w1785 w1793 w1834 w1840 w1886 w1919 w1993 w2062 w2147 w2195 w2242]
      tunnel: w65 -> [_ _ _ _ _ _ _ _ _ _ _ _ _ _ _ _ w751 _ _ _ _ _ _ _ _ _ _ _ _ _ w1182 w1351 _ _ w1589 _ w1704 _ _ w1792 _ _ _ _ _ _ _ _ _]
      tunnel: w64 -> [_ _ _ _ _ _ _ _ _ _ _ _ _ _ _ _ _ _ _ _ _ _ _ _ _ _ _ _ _ _ w1179 _ _ _ _ _ _ _ _ _ _ _ _ _ _ _ _ _ _]
      tunnel: w63 -> [w83 w86 w92 w95 w200 w222 w239 w243 w299 w345 w395 w411 w455 w495 w564 w662 w754 w814 w870 w921 w931 w938 w943 w946 w988 w997 w1037 w1072 w1117 w1151 w1178 w1346 w1448 w1523 w1592 w1649 w1699 w1734 w1784 w1788 w1833 w1839 w1882 w1915 w1989 w2058 w2144 w2191 w2241]
      tunnel: [w83 w86 w92 w95 w200 w222 w239 w242 w298 w344 w395 w410 w454 w494 w563 w661 w753 w813 w869 w921 w931 w938 w943 w945 w987 w996 w1036 w1071 w1116 w1150 w1175 w1345 w1447 w1522 w1591 w1648 w1698 w1733 w1784 w1787 w1833 w1838 w1881 w1914 w1988 w2057 w2143 w2190 w2238] -> w62
      tunnel: [_ _ _ _ _ _ _ _ _ _ _ _ _ _ _ _ _ _ _ _ _ _ _ TRUE _ _ _ _ _ _ _ _ _ _ _ _ _ _ _ _ _ _ _ _ _ _ _ _ _] -> w57
      tunnel: w52 -> [_ _ _ _ _ _ _ _ _ _ _ _ _ _ _ _ _ _ _ _ _ _ _ _ _ _ _ _ _ _ _ w1340 _ _ _ _ _ _ _ _ _ _ _ _ _ _ _ _ _]
      tunnel: w51 -> [_ _ _ w104 _ _ _ _ _ _ _ _ _ _ _ _ w750 _ _ _ _ _ _ _ _ _ _ _ _ _ w1174 w1339 _ _ w1588 _ _ _ _ w1786 _ _ _ _ _ _ _ _ _]
      tunnel: w45 -> [_ _ _ _ _ _ _ _ _ _ _ _ _ _ _ _ _ _ _ _ w930 _ _ _ _ _ _ _ _ _ _ _ _ _ _ _ _ _ _ _ _ _ _ _ _ _ _ _ _]
      tunnel: w44 -> [_ _ _ w103 _ _ _ _ _ _ _ _ _ _ w559 _ _ _ _ _ _ _ _ _ _ _ _ _ _ _ _ _ w1445 _ _ _ _ _ _ _ _ _ _ _ _ _ _ _ _]
      tunnel: w43 -> [_ _ _ _ _ _ _ _ _ _ _ _ _ _ _ _ _ _ _ _ _ _ _ _ _ _ _ _ _ _ _ _ _ _ _ _ _ _ _ _ _ _ _ _ _ _ _ _ _]
      frame "<--------------- Application ONLY --------------->" {
      }
      frame Default {
        n22 = Concatenate Strings(w87, " Not a Valid Command" ("string")) -> (w88:string)
        n23 = call <vilib>:"NI VeriStand - Print Debug String.vi"("Message"=w88) -> ()  [unwired: 10 in, 1 out]
      }
      frame "RestartCANComm" {
      }
      frame "", "CheckPoll" {
        n24 = Unbundle By Name(w100) -> ("Polling.Enabled"=w99:bool[], "Polling.Queued"=w96:bool[], "Polling.Last Generation"=w102:u32[])
        n25 = Or Array Elements(Boolean array=w99) -> (logical OR=w98:bool)
        n26 = case shown="True" w98 {
          tunnel: [w110 w120] -> w107
          tunnel: w106 -> [w109 w119]
          tunnel: [w109 w118] -> w105
          tunnel: w104 -> [_ w117]
          tunnel: w103 -> [_ w116]
          tunnel: w102 -> [w110 w115]
          tunnel: w99 -> [_ w114]
          tunnel: w96 -> [w108 w112]
          tunnel: [w108 w111] -> w97
          frame False {
          }
          frame True {
            n27 = call "Tick Count2"() -> ("Tick Count(mSec)"=w113:u32)
            n28 = for {
              tunnel: w116 -> [w137] mode=indexing
              tunnel: w115 -> [w125] mode=indexing
              tunnel: [w138] -> w120 mode=indexing
              shift-right: [w133] -> w118
              shift-left: w119 -> [w134]
              tunnel: w117 -> [w132]
              tunnel: w114 -> [w124] mode=indexing
              tunnel: w113 -> [w131]
              tunnel: w112 -> [w123] mode=indexing
              tunnel: [w128] -> w111 mode=indexing
              i -> [w127]
              n29 = Unbundle By Name(w137) -> ("Speed"=w136:T15, "DID IDs"=w129:u32[], "PID IDs"=w130:u32[])
              n30 = Subtract(x=w131, y=w125) -> (x-y=w126:u32)
              n31 = To Unsigned Long Integer(number=w127) -> (unsigned 32bit integer=w122:u32)
              n32 = case shown="\"Slow\"" w136 {
                tunnel: [u32 1000 ("Tick Count(mSec)") u32 50 ("Tick Count(mSec)") u32 100 ("Tick Count(mSec)")] -> w121
                frame "Slow" {
                }
                frame "Fast" {
                }
                frame "Medium" {
                }
              }
              n33 = Greater Or Equal?(x=w126, y=w121) -> (x >= y?=w135:bool)
              n34 = case shown="True" w124 {
                tunnel: w125 -> [w139 w154]
                tunnel: [w139 w153] -> w138
                tunnel: w131 -> [_ w152]
                tunnel: w135 -> [_ w144]
                tunnel: w134 -> [w141 w151]
                tunnel: [w141 w150] -> w133
                tunnel: w132 -> [_ w149]
                tunnel: w130 -> [_ w148]
                tunnel: w129 -> [_ w147]
                tunnel: w122 -> [_ w146]
                tunnel: w123 -> [_ w142]
                tunnel: [FALSE w143] -> w128
                frame False {
                }
                frame True {
                  n35 = Compound Arithmetic op=AND(invert w142, w144) -> (w145:bool)
                  n36 = case shown="True" w145 {
                    tunnel: w152 -> [_ w160]
                    tunnel: w154 -> [w155 _]
                    tunnel: [w155 w160] -> w153
                    tunnel: w151 -> [w157 w164]
                    tunnel: [w157 w171] -> w150
                    tunnel: w149 -> [_ w168]
                    tunnel: w148 -> [_ w170]
                    tunnel: w147 -> [_ w169]
                    tunnel: w146 -> [_ w158]
                    tunnel: [w156 TRUE] -> w143
                    tunnel: w142 -> [w156 _]
                    frame False {
                    }
                    frame True {
                      n37 = Empty Array?(array=w169) -> (empty?=w167:bool)
                      n38 = Flatten To String(anything=w158, error in (no error)=w164) -> (data string=w159:string, error out=w163:errorcluster)  [unwired: 2 in, 1 out]
                      n39 = Empty Array?(array=w170) -> (empty?=w166:bool)
                      n40 = case shown="False" w167 {
                        tunnel: w166 -> [w175 w185]
                        tunnel: [w174 w184] -> w165
                        tunnel: w159 -> [w173 w183]
                        tunnel: [w172 w182] -> w162
                        frame False {
                          n41 = case shown="True" w175 {
                            tunnel: [string[] ["PollDIDs", "PollPIDs"] ("message names") string[] ["PollDIDs"] ("message names")] -> w174
                            tunnel: w173 -> [w177 w180]
                            tunnel: [w176 w179] -> w172
                            frame False {
                              n42 = Build Array(w177, w177) -> (w176:string[])
                            }
                            frame True {
                              n43 = Build Array(w180) -> (w179:string[])
                            }
                          }
                        }
                        frame True {
                          n44 = case shown="False" w185 {
                            tunnel: [string[] ["PollPIDs"] ("message names") _] -> w184
                            tunnel: w183 -> [w187 _]
                            tunnel: [w186 _] -> w182
                            frame False {
                              n45 = Build Array(w187) -> (w186:string[])
                            }
                            frame True {
                            }
                          }
                        }
                      }
                      n46 = call <vilib>:"Send Commands.vi"("error in (no error)"=w163, "message values"=w162, "message names"=w165, "VeriStand Comm in"=w168) -> ("error out"=w171:errorcluster)  [unwired: 6 in, 1 out]
                    }
                  }
                }
              }
            }
          }
        }
        n47 = Bundle By Name(cluster=w100, "Polling.Queued"=w97, "Polling.Last Generation"=w107) -> (w101:T31)
      }
      frame "StopPolling" {
        n48 = Unflatten From String(type=u32 0, binary string=w195, error in (no error)=w193) -> (value=w192:u32, error out=w194:errorcluster)  [unwired: 2 in, 1 out]
        n49 = case shown="0" w192 {
          selector: w192 -> [_ w208]
          tunnel: w197 -> [w206 w213]
          tunnel: [w203 w212] -> w198
          tunnel: FALSE -> [w202 w210]
          frame 0 {
            n50 = Unbundle By Name(w206) -> ("Polling.Enabled"=w205:bool[])
            n51 = Array Size(array=w205) -> (size(s)=w204:i32)
            n52 = Initialize Array(w202, w204) -> (w201:bool[])
            n53 = Bundle By Name(cluster=w206, "Polling.Enabled"=w201, "Polling.Queued"=w201) -> (w203:T31)
          }
          frame Default {
            n54 = Unbundle By Name(w213) -> ("Polling.Enabled"=w211:bool[])
            n55 = Decrement(x=w208) -> (x-1=w207:u32)
            n56 = Replace Array Subset(array=w211, new element=w210, index=w207) -> (w209:bool[])
            n57 = Bundle By Name(cluster=w213, "Polling.Enabled"=w209) -> (w212:T31)
          }
        }
      }
      frame "StartPolling" {
        n58 = Unflatten From String(type=u32 0, binary string=w217, error in (no error)=w215) -> (value=w214:u32, error out=w216:errorcluster)  [unwired: 2 in, 1 out]
        n59 = case shown="0" w214 {
          selector: w214 -> [_ w232]
          tunnel: w219 -> [w230 w237]
          tunnel: [w227 w236] -> w220
          tunnel: TRUE -> [w226 w234]
          frame 0 {
            n60 = Unbundle By Name(w230) -> ("Polling.Enabled"=w229:bool[])
            n61 = Array Size(array=w229) -> (size(s)=w225:i32)
            n62 = Initialize Array(w226, w225) -> (w228:bool[])
            n63 = Initialize Array(FALSE ("element"), w225) -> (w223:bool[])
            n64 = Bundle By Name(cluster=w230, "Polling.Enabled"=w228, "Polling.Queued"=w223) -> (w227:T31)
          }
          frame Default {
            n65 = Unbundle By Name(w237) -> ("Polling.Enabled"=w235:bool[])
            n66 = Decrement(x=w232) -> (x-1=w231:u32)
            n67 = Replace Array Subset(array=w235, new element=w234, index=w231) -> (w233:bool[])
            n68 = Bundle By Name(cluster=w237, "Polling.Enabled"=w233) -> (w236:T31)
          }
        }
      }
      frame "<--------------- GMLAN ONLY --------------->" {
      }
      frame "DTCCountChanged", "StartDTCs" {
        n69 = in-place {
          in-place-border: w248 -> [w259]
          in-place-border: [w258] -> w247
          in-place-border: w246 -> [w257]
          in-place-border: w245 -> [w256]
          n70 = in-place-cluster #1(w243) -> ("Status"=w251:T26, "ADCS Connection"=w254:T19, "Parameters.Properties.CAN.Diagnostic Protocol"=w252:T6)
          n71 = in-place-cluster #2(w244) -> ("status mask"=w255:u8)
          n72 = case shown="\"GMLAN\"" w252 {
            selector: w252 -> [w260 w264]
            tunnel: w259 -> [w261 w278]
            tunnel: [w261 w277] -> w258
            tunnel: w257 -> [_ w276]
            tunnel: w256 -> [_ w275]
            tunnel: w255 -> [_ w274]
            tunnel: w254 -> [w263 w272]
            tunnel: [w263 w269] -> w253
            tunnel: w251 -> [w262 w265]
            tunnel: [w262 w265] -> w250
            tunnel: [w260 w264] -> w249
            frame Default {
            }
            frame "GMLAN" {
              w286 = Property_ID."Timeout Diag Command" ("property ID")
              n73 = case shown="Default" w276 {
                tunnel: w278 -> [w290 w295]
                tunnel: w275 -> [_ w294]
                tunnel: [w289 w292] -> w281
                tunnel: [w290 w291] -> w284
                tunnel: w274 -> [w289 _]
                frame "DTCCountChanged" {
                }
                frame Default {
                  n74 = Unflatten From String(type=u8 0 ("status mask"), binary string=w294, error in (no error)=w295) -> (value=w292:u8, error out=w291:errorcluster)  [unwired: 2 in, 1 out]
                }
              }
              n75 = Number To Boolean Array(number=w281) -> (Boolean array=w280:bool[])
              n76 = Array To Cluster(array=w280) -> (cluster=w279:T51)
              n77 = call <vilib>:"Diag Get Property.vi"("error in (no error)"=w284, "property ID"=w286, "diag ref in"=w272) -> ("error out"=w288:errorcluster, "property value"=w282:u32, "diag ref out"=w273:T19)  [unwired: 6 in]
              n78 = call <vilib>:"Diag Set Property.vi"("error in (no error)"=w288, "property value"=u32 100, "property ID"=w286, "diag ref in"=w273) -> ("error out"=w283:errorcluster, "diag ref out"=w271:T19)  [unwired: 6 in]
              n79 = call "ReadDiagnosticInformation_ByStatus.vi"("error in (no error)"=w283, "status mask"=w279, "diag ref in"=w271) -> ("error out"=w268:errorcluster, "success?"=w267:bool, "diag ref out"=w270:T19)  [unwired: 5 in, 1 out]
              n80 = call "Status.Set.vi"("error in (no error)"=w268, "success?"=w267, "Status Ref"=w265) -> ("error out"=w266:errorcluster)  [unwired: 8 in]
              n81 = call <vilib>:"Diag Set Property.vi"("error in (no error)"=w266, "property value"=w282, "property ID"=Property_ID."Timeout Diag Command", "diag ref in"=w270) -> ("error out"=w277:errorcluster, "diag ref out"=w269:T19)  [unwired: 6 in]
            }
          }
          n82 = in-place-cluster #1("Status"=w250, "ADCS Connection"=w253, "Parameters.Properties.CAN.Diagnostic Protocol"=w249) -> (w242:T1)
          n83 = in-place-cluster #2("status mask"=w255) -> (w241:T31)
        }
      }
      frame "DisableChangeDTCCount", "EnableChangeDTCCount" {
        n84 = in-place {
          in-place-border: w302 -> [w313]
          in-place-border: [w312] -> w301
          in-place-border: w300 -> [w311]
          n85 = in-place-cluster #3(w299) -> ("Status"=w307:T26, "ADCS Connection"=w309:T19, "Parameters.Properties.CAN.Diagnostic Protocol"=w304:T6)
          n86 = in-place-cluster #4(w297) -> ("status mask"=w306:u8)
          n87 = case shown="\"GMLAN\"" w304 {
            selector: w304 -> [w314 w319]
            tunnel: w313 -> [w317 w333]
            tunnel: [w317 w332] -> w312
            tunnel: w311 -> [_ w331]
            tunnel: [w318 w330] -> w310
            tunnel: w309 -> [w316 w328]
            tunnel: [w316 w325] -> w308
            tunnel: w307 -> [w315 w320]
            tunnel: w306 -> [w318 _]
            tunnel: [w315 w320] -> w305
            tunnel: [w314 w319] -> w303
            frame Default {
            }
            frame "GMLAN" {
              w340 = Property_ID."Timeout Diag Command" ("property ID")
              n88 = Unflatten From String(type=u8 0 ("status mask"), binary string=w331, error in (no error)=w333) -> (value=w330:u8, error out=w338:errorcluster)  [unwired: 2 in, 1 out]
              n89 = Number To Boolean Array(number=w330) -> (Boolean array=w335:bool[])
              n90 = Array To Cluster(array=w335) -> (cluster=w334:T51)
              n91 = call <vilib>:"Diag Get Property.vi"("error in (no error)"=w338, "property ID"=w340, "diag ref in"=w328) -> ("error out"=w342:errorcluster, "property value"=w336:u32, "diag ref out"=w329:T19)  [unwired: 6 in]
              n92 = call <vilib>:"Diag Set Property.vi"("error in (no error)"=w342, "property value"=u32 100, "property ID"=w340, "diag ref in"=w329) -> ("error out"=w337:errorcluster, "diag ref out"=w327:T19)  [unwired: 6 in]
              n93 = call "ReadDiagnosticInformation_sendOnChangeDTCCount.vi"("error in (no error)"=w337, "status mask"=w334, "diag ref in"=w327) -> ("error out"=w324:errorcluster, "success?"=w321:bool, "data out"=w322:u8[], "diag ref out"=w326:T19)  [unwired: 5 in]
              n94 = call "Status.Set.vi"("error in (no error)"=w324, "success?"=w321, "Data"=w322, "Status Ref"=w320) -> ("error out"=w323:errorcluster)  [unwired: 7 in]
              n95 = call <vilib>:"Diag Set Property.vi"("error in (no error)"=w323, "property value"=w336, "property ID"=Property_ID."Timeout Diag Command", "diag ref in"=w326) -> ("error out"=w332:errorcluster, "diag ref out"=w325:T19)  [unwired: 6 in]
            }
          }
          n96 = in-place-cluster #3("Status"=w305, "ADCS Connection"=w308, "Parameters.Properties.CAN.Diagnostic Protocol"=w303) -> (w298:T1)
          n97 = in-place-cluster #4("status mask"=w310) -> (w296:T31)
        }
      }
      frame "ReadFailureRecordParameters" {
        n98 = in-place {
          in-place-border: w348 -> [w358]
          in-place-border: w347 -> [w357]
          in-place-border: [w356] -> w346
          n99 = in-place-cluster #5(w345) -> ("Status"=w353:T26, "ADCS Connection"=w355:T19, "Parameters.Properties.CAN.Diagnostic Protocol"=w351:T6)
          n100 = case shown="\"GMLAN\"" w351 {
            selector: w351 -> [w360 w363]
            tunnel: w358 -> [_ w376]
            tunnel: w357 -> [w359 w375]
            tunnel: [w359 w374] -> w356
            tunnel: w355 -> [w361 w372]
            tunnel: [w361 w369] -> w354
            tunnel: w353 -> [w362 w364]
            tunnel: [w362 w364] -> w352
            tunnel: [w360 w363] -> w350
            frame Default {
            }
            frame "GMLAN" {
              w391 = Property_ID."Timeout Diag Command" ("property ID")
              n101 = Unflatten From String(type=T33 {"failureRecordNumber"=0, "DTC ID"=0, "DTCFailureType"=0} ("failureRecordIdentifier"), binary string=w376, error in (no error)=w375) -> (value=w377:T33, error out=w389:errorcluster)  [unwired: 2 in, 1 out]
              n102 = call <vilib>:"Diag Get Property.vi"("error in (no error)"=w389, "property ID"=w391, "diag ref in"=w372) -> ("error out"=w393:errorcluster, "property value"=w387:u32, "diag ref out"=w373:T19)  [unwired: 6 in]
              n103 = call <vilib>:"Diag Set Property.vi"("error in (no error)"=w393, "property value"=u32 1000, "property ID"=w391, "diag ref in"=w373) -> ("error out"=w388:errorcluster, "diag ref out"=w371:T19)  [unwired: 6 in]
              n104 = call "ReadFailureRecordData_readFailureRecordParameters.vi"("error in (no error)"=w388, "failureRecordIdentifier"=w377, "diag ref in"=w371) -> ("error out"=w367:errorcluster, "success?"=w368:bool, "data out"=w365:u8[], "diag ref out"=w370:T19)  [unwired: 5 in]
              n105 = Open/Create/Replace File(file path (use dialog)=path "C:/ReadFailureRecordParameters.txt", operation (0:open)=T34."replace or create") -> (refnum out=w381:refnum<file>, error out=w384:errorcluster)  [unwired: 4 in, 1 out]
              n106 = Array To Spreadsheet String(array=w365, 3:"%x" ("format string")) -> (spreadsheet string=w379:string)  [unwired: 1 in]
              n107 = Write to Text File(file (use dialog)=w381, text=w379, error in=w384) -> (refnum out=w380:refnum<file>, error out=w383:errorcluster)  [unwired: 1 in, 1 out]
              n108 = Close File(refnum=w380, error in=w383) -> ()  [unwired: 2 out]
              n109 = call "Status.Set.vi"("error in (no error)"=w367, "success?"=w368, "Data"=w365, "Status Ref"=w364) -> ("error out"=w366:errorcluster)  [unwired: 7 in]
              n110 = call <vilib>:"Diag Set Property.vi"("error in (no error)"=w366, "property value"=w387, "property ID"=Property_ID."Timeout Diag Command", "diag ref in"=w370) -> ("error out"=w374:errorcluster, "diag ref out"=w369:T19)  [unwired: 6 in]
            }
          }
          n111 = in-place-cluster #5("Status"=w352, "ADCS Connection"=w354, "Parameters.Properties.CAN.Diagnostic Protocol"=w350) -> (w344:T1)
        }
      }
      frame "UpdateDTCReport" {
        n112 = Unbundle By Name(w395) -> ("Parameters.Properties.CAN.Diagnostic Protocol"=w394:T6)
        n113 = case shown="\"GMLAN\"" w394 {
          tunnel: w400 -> [w402 w407]
          tunnel: [w402 w406] -> w399
          tunnel: w396 -> [w401 w405]
          tunnel: [w401 w404] -> w398
          tunnel: w397 -> [_ w403]
          frame Default {
          }
          frame "GMLAN" {
            n114 = Unflatten From String(type=T30[] [] ("Active DTCs"), binary string=w403, error in (no error)=w407) -> (value=w409:T30[], error out=w406:errorcluster)  [unwired: 2 in, 1 out]
            n115 = Bundle By Name(cluster=w405, "Active DTCs"=w409) -> (w404:T31)
          }
        }
      }
      frame "ReadDTCByDTCNumber" {
        n116 = in-place {
          in-place-border: w414 -> [w424]
          in-place-border: w413 -> [w423]
          in-place-border: [w422] -> w412
          n117 = in-place-cluster #6(w411) -> ("Status"=w419:T26, "ADCS Connection"=w421:T19, "Parameters.Properties.CAN.Diagnostic Protocol"=w416:T6)
          n118 = case shown="\"GMLAN\"" w416 {
            selector: w416 -> [w427 w429]
            tunnel: w424 -> [_ w442]
            tunnel: w423 -> [w428 w441]
            tunnel: [w428 w440] -> w422
            tunnel: w421 -> [w426 w438]
            tunnel: [w426 w435] -> w420
            tunnel: w419 -> [w425 w430]
            tunnel: [w427 w429] -> w418
            tunnel: [w425 w430] -> w417
            frame Default {
            }
            frame "GMLAN" {
              w451 = Property_ID."Timeout Diag Command" ("property ID")
              n119 = Unflatten From String(type=T35 {"DTC"=0, "FailTypeByte"=0}, binary string=w442, error in (no error)=w441) -> (value=w445:T35, error out=w449:errorcluster)  [unwired: 2 in, 1 out]
              n120 = Unbundle By Name(w445) -> ("DTC"=w444:u16, "FailTypeByte"=w443:u8)
              n121 = call <vilib>:"Diag Get Property.vi"("error in (no error)"=w449, "property ID"=w451, "diag ref in"=w438) -> ("error out"=w453:errorcluster, "property value"=w447:u32, "diag ref out"=w439:T19)  [unwired: 6 in]
              n122 = call <vilib>:"Diag Set Property.vi"("error in (no error)"=w453, "property value"=u32 100, "property ID"=w451, "diag ref in"=w439) -> ("error out"=w448:errorcluster, "diag ref out"=w437:T19)  [unwired: 6 in]
              n123 = call "ReadDiagnosticInformation_readStatusOfDTCByDTCNumber.vi"("error in (no error)"=w448, "FailTypeByte"=w443, "DTC"=w444, "diag ref in"=w437) -> ("error out"=w432:errorcluster, "success?"=w433:bool, "data out"=w434:u8[], "diag ref out"=w436:T19)  [unwired: 4 in]
              n124 = call "Status.Set.vi"("error in (no error)"=w432, "success?"=w433, "Data"=w434, "Status Ref"=w430) -> ("error out"=w431:errorcluster)  [unwired: 7 in]
              n125 = call <vilib>:"Diag Set Property.vi"("error in (no error)"=w431, "property value"=w447, "property ID"=Property_ID."Timeout Diag Command", "diag ref in"=w436) -> ("error out"=w440:errorcluster, "diag ref out"=w435:T19)  [unwired: 6 in]
            }
          }
          n126 = in-place-cluster #6("Status"=w417, "ADCS Connection"=w420, "Parameters.Properties.CAN.Diagnostic Protocol"=w418) -> (w410:T1)
        }
      }
      frame "ConfigurePIDs" {
        n127 = in-place {
          in-place-border: w457 -> [w468]
          in-place-border: [w464] -> w456
          n128 = in-place-cluster #7(w455) -> ("Status"=w463:T26, "Parameters.Properties.DPIDs"=w467:T14[], "ADCS Connection"=w466:T19, "Parameters.Properties.CAN.Diagnostic Protocol"=w462:T6)
          n129 = case shown="\"GMLAN\"" w462 {
            selector: w462 -> [w473 w476]
            tunnel: w468 -> [w471 w483]
            tunnel: w467 -> [w469 w475]
            tunnel: w466 -> [w472 w481]
            tunnel: [w472 w480] -> w465
            tunnel: [w471 w477] -> w464
            tunnel: w463 -> [w470 w474]
            tunnel: [w473 w476] -> w461
            tunnel: [w470 w474] -> w460
            tunnel: [w469 w475] -> w459
            frame Default {
            }
            frame "GMLAN" {
              n130 = for {
                shift-right: [w490] -> w480
                shift-left: w481 -> [w491]
                tunnel: w475 -> [w489] mode=indexing
                shift-right: [w485] -> w478
                shift-left: w483 -> [w486]
                tunnel: [w484] -> w482 mode=indexing
                n131 = Unbundle By Name(w489) -> ("DPID ID"=w488:u8, "PIDs"=w487:u16[])
                n132 = call "GMLAN DynamicallyDefineMessage.vi"("error in (no error)"=w486, "PID List"=w487, "DPID ID"=w488, "diag ref in"=w491) -> ("error out"=w485:errorcluster, "success?"=w484:bool, "diag ref out"=w490:T19)  [unwired: 5 in]
              }
              n133 = And Array Elements(Boolean array=w482) -> (logical AND=w479:bool)
              n134 = call "Status.Set.vi"("error in (no error)"=w478, "success?"=w479, "Status Ref"=w474) -> ("error out"=w477:errorcluster)  [unwired: 8 in]
            }
          }
          n135 = in-place-cluster #7("Status"=w460, "Parameters.Properties.DPIDs"=w459, "ADCS Connection"=w465, "Parameters.Properties.CAN.Diagnostic Protocol"=w461) -> (w454:T1)
        }
      }
      frame "StartPIDs" {
        n136 = in-place {
          in-place-border: w493 -> [w506]
          in-place-border: [w505] -> w492
          n137 = in-place-cluster #8(w495) -> ("Status"=w501:T26, "ADCS Connection"=w503:T19, "Parameters.Properties.DPIDs"=w504:T14[], "Parameters.Properties.CAN.Diagnostic Protocol"=w500:T6)
          n138 = case shown="\"GMLAN\"" w500 {
            selector: w500 -> [w509 w514]
            tunnel: w506 -> [w511 w527]
            tunnel: [w511 w525] -> w505
            tunnel: w504 -> [w510 w513]
            tunnel: w503 -> [w508 w521]
            tunnel: [w508 w518] -> w502
            tunnel: w501 -> [w507 w512]
            tunnel: [w509 w514] -> w499
            tunnel: [w510 w513] -> w498
            tunnel: [w507 w512] -> w497
            frame Default {
            }
            frame "GMLAN" {
              w529 = Property_ID."Timeout Diag Command" ("property ID")
              w533 = T37[] [enum."scheduleAtSlowRate", enum."scheduleAtMediumRate", enum."scheduleAtFastRate"] items=["stopSending", "sendOneResponse", "scheduleAtSlowRate", "scheduleAtMediumRate", "scheduleAtFastRate"]
              n139 = call <vilib>:"Diag Get Property.vi"("error in (no error)"=w527, "property ID"=w529, "diag ref in"=w521) -> ("error out"=w531:errorcluster, "property value"=w524:u32, "diag ref out"=w522:T19)  [unwired: 6 in]
              n140 = call <vilib>:"Diag Set Property.vi"("error in (no error)"=w531, "property value"=u32 100, "property ID"=w529, "diag ref in"=w522) -> ("error out"=w526:errorcluster, "diag ref out"=w520:T19)  [unwired: 6 in]
              n141 = call "DPIDs.IDs.Sort.vi"("DPIDs"=w513) -> ("Filtered DPIDs IDs"=w532:T52)  [unwired: 10 in]
              n142 = for {
                tunnel: w532 -> [w539]
                shift-right: [w534] -> w516
                shift-left: w526 -> [w542]
                shift-right: [w540] -> w519
                shift-left: w520 -> [w541]
                tunnel: w533 -> [w536] mode=indexing
                tunnel: [w535] -> w523 mode=indexing
                stop <- w534 stop-if-true
                n143 = case shown="\"scheduleAtFastRate\"" w536 {
                  tunnel: w539 -> [w554 w556 _ w558]
                  tunnel: [w553 w555 _ w557] -> w538
                  frame "scheduleAtMediumRate" {
                    n144 = Unbundle By Name(w554) -> ("Medium"=w553:u8[])
                  }
                  frame "scheduleAtFastRate" {
                    n145 = Unbundle By Name(w556) -> ("Fast"=w555:u8[])
                  }
                  frame Default {
                  }
                  frame "scheduleAtSlowRate" {
                    n146 = Unbundle By Name(w558) -> ("Slow"=w557:u8[])
                  }
                }
                n147 = Empty Array?(array=w538) -> (empty?=w537:bool)
                n148 = case shown="False" w537 {
                  tunnel: w542 -> [w549 w551]
                  tunnel: [w548 w551] -> w534
                  tunnel: w541 -> [w547 w552]
                  tunnel: [w546 w552] -> w540
                  tunnel: w536 -> [w543 _]
                  tunnel: w538 -> [w545 _]
                  tunnel: [w544 TRUE ("success?")] -> w535
                  frame False {
                    n149 = call "GMLAN ReadDataByPacketIdentifier.vi"("error in (no error)"=w549, "DPIDs"=w545, "Sub Function"=w543, "diag ref in"=w547) -> ("error out"=w548:errorcluster, "success?"=w544:bool, "diag ref out"=w546:T19)  [unwired: 4 in, 1 out]
                  }
                  frame True {
                  }
                }
              }
              n150 = And Array Elements(Boolean array=w523) -> (logical AND=w517:bool)
              n151 = call "Status.Set.vi"("error in (no error)"=w516, "success?"=w517, "Status Ref"=w512) -> ("error out"=w515:errorcluster)  [unwired: 8 in]
              n152 = call <vilib>:"Diag Set Property.vi"("error in (no error)"=w515, "property value"=w524, "property ID"=Property_ID."Timeout Diag Command", "diag ref in"=w519) -> ("error out"=w525:errorcluster, "diag ref out"=w518:T19)  [unwired: 6 in]
            }
          }
          n153 = in-place-cluster #8("Status"=w497, "ADCS Connection"=w502, "Parameters.Properties.DPIDs"=w498, "Parameters.Properties.CAN.Diagnostic Protocol"=w499) -> (w494:T1)
        }
      }
      frame "PollPIDs" {
        n154 = in-place {
          in-place-border: w566 -> [w571]
          in-place-border: [w578] -> w565
          in-place-border: w560 -> [w570]
          in-place-border: w559 -> [w569]
          n155 = in-place-cluster #9(w562) -> ("Polling.Queued"=w573:bool[])
          n156 = in-place-cluster #10(w564) -> ("Status"=w588:T26, "Parameters.Properties.Service Channels Status Lookup"=w583:variant, "Service Channels Status"=w580:T26, "Parameters.Properties.Frames Lookup"=w592:variant, "Reads"=w581:T26, "XNETEngine (GMLAN)"=w590:T25, "ADCS Connection"=w585:T19, "Parameters.Properties.CAN.Diagnostic Protocol"=w591:T6)
          n157 = Unflatten From String(type=u32 0 ("ID"), binary string=w570, error in (no error)=w571) -> (value=w575:u32, error out=w568:errorcluster)  [unwired: 2 in, 1 out]
          n158 = Index Array(array=w569, index=w575) -> (element=w576:T18)
          n159 = Replace Array Subset(array=w573, new element=FALSE ("new element/subarray"), index=w575) -> (w572:bool[])
          n160 = Unbundle By Name(w576) -> ("PID IDs"=w567:u32[])
          n161 = case shown="\"GMLAN\"" w591 {
            tunnel: [w608 w659] -> w587
            tunnel: [w604 _] -> w593
            tunnel: w568 -> [w609 w659]
            tunnel: w567 -> [w606 _]
            tunnel: w592 -> [w601 _]
            tunnel: w585 -> [w607 w658]
            tunnel: [w605 w658] -> w584
            tunnel: w590 -> [w603 _]
            tunnel: [w602 _] -> w586
            tunnel: w581 -> [w600 _]
            tunnel: w580 -> [w599 _]
            tunnel: w583 -> [w598 _]
            frame "GMLAN" {
              n162 = disable-structure shown="InlinePID==FALSE, Default" {
                disable-tunnel: w609 -> [w617 w642]
                disable-tunnel: [w616 w632] -> w608
                disable-tunnel: w607 -> [w615 w641]
                disable-tunnel: w606 -> [w614 w640]
                disable-tunnel: [w613 w639] -> w605
                disable-tunnel: [w612 w638] -> w604
                disable-tunnel: w603 -> [w611 _]
                disable-tunnel: [w610 w637] -> w602
                disable-tunnel: w601 -> [_ w636]
                disable-tunnel: w600 -> [_ w635]
                disable-tunnel: w599 -> [_ w634]
                disable-tunnel: w598 -> [_ w633]
                frame condition #0 {
                  n163 = for {
                    shift-right: [w623] -> w622
                    shift-left: w617 -> [w631]
                    shift-right: [w629] -> w613
                    shift-left: w615 -> [w630]
                    tunnel: w614 -> [w625] mode=indexing
                    tunnel: [w628] -> w612 mode=indexing
                    tunnel: [w627] -> w618 mode=indexing
                    tunnel: [w624] -> w610
                    stop <- w623 stop-if-true
                    n164 = call "GMLAN ReadDataByParameterIdentifier.vi"("error in (no error)"=w631, "Parameter ID (PID)"=w625, "diag ref in"=w630) -> ("error out"=w623:errorcluster, "success?"=w628:bool, "data out"=w624:u8[], "diag ref out"=w629:T19)  [unwired: 5 in]
                    n165 = Bundle By Name(cluster=T36 {"ID"=0, "Raw Frame"=[], "error out"={"status"=FALSE, "code"=0, "source"=""}}, "ID"=w625, "Raw Frame"=w624, "error out"=w623) -> (w627:T36)
                  }
                  n166 = Flatten To String(anything=w618, error in (no error)=w622) -> (data string=w619:string, error out=w621:errorcluster)  [unwired: 2 in, 1 out]
                  n167 = call <vilib>:"Send Local Message.vi"("message queue in"=w611, "message name"="UpdatePIDsOnDemand" ("Message Name"), "message value"=w619, "error in"=w621) -> ("error out"=w616:errorcluster)  [unwired: 9 in, 2 out]
                }
                frame condition #1 (active) {
                  n168 = for {
                    shift-right: [w650] -> w632
                    shift-left: w642 -> [w657]
                    shift-right: [w655] -> w639
                    shift-left: w641 -> [w656]
                    tunnel: w640 -> [w649] mode=indexing
                    tunnel: [w654] -> w638 mode=indexing
                    tunnel: [w648] -> w637
                    tunnel: w636 -> [w647]
                    tunnel: w635 -> [w646]
                    tunnel: w634 -> [w645]
                    tunnel: w633 -> [w644]
                    stop <- w650 stop-if-true
                    w643 = TRUE ("Buffer?")
                    w652 = Type."PID" ("Type")
                    n169 = call "GMLAN ReadDataByParameterIdentifier.vi"("error in (no error)"=w657, "Parameter ID (PID)"=w649, "diag ref in"=w656) -> ("error out"=w651:errorcluster, "success?"=w654:bool, "data out"=w648:u8[], "diag ref out"=w655:T19)  [unwired: 5 in]
                    n170 = call "Signals.Scale.EU.vi"("Buffer?"=w643, "Type"=w652, "Lookup"=w647, "error in (no error)"=w651, "Unscaled Data"=w648, "ID"=w649, "Reads Ref"=w646) -> ("error out"=w653:errorcluster)  [unwired: 4 in]
                    n171 = call "ServiceChannels.Status.Set.vi"("Buffer?"=w643, "Type"=w652, "Status Lookup"=w644, "error in (no error)"=w653, "ID"=w649, "Service Channels Status Ref"=w645) -> ("error out"=w650:errorcluster)  [unwired: 5 in]
                  }
                }
              }
            }
            frame "KWP-2000".."User-Defined" {
            }
          }
          n172 = And Array Elements(Boolean array=w593) -> (logical AND=w589:bool)
          n173 = call "Status.Set.vi"("error in (no error)"=w587, "success?"=w589, "Data"=w586, "Status Ref"=w588) -> ("error out"=w582:errorcluster)  [unwired: 7 in]
          n174 = call-poly <vilib>:"Data.Processes.Execute.vi"("error in (no error)"=w582, "Ref"=w581) -> ("error out"=w579:errorcluster)  [unwired: 9 in]
          n175 = flat-sequence {
            tunnel: w580 -> [w597]
            tunnel: w579 -> [w596]
            tunnel: [w594] -> w578
            frame #0 {
              n176 = call-poly <vilib>:"Data.Processes.Execute.vi"("Ref"=w597) -> ("error out"=w595:errorcluster)  [unwired: 10 in]
              n177 = Merge Errors(w596, w595) -> (w594:errorcluster)
            }
          }
          n178 = in-place-cluster #10("Status"=w588, "Parameters.Properties.Service Channels Status Lookup"=w583, "Service Channels Status"=w580, "Parameters.Properties.Frames Lookup"=w592, "Reads"=w581, "XNETEngine (GMLAN)"=w590, "ADCS Connection"=w584, "Parameters.Properties.CAN.Diagnostic Protocol"=w591) -> (w563:T1)
          n179 = in-place-cluster #9("Polling.Queued"=w572) -> (w561:T31)
        }
      }
      frame "ReadPIDsOnDemand" {
        n180 = in-place {
          in-place-border: w664 -> [w682]
          in-place-border: [w665] -> w663
          in-place-border: w660 -> [w678]
          n181 = in-place-cluster #11(w662) -> ("Status"=w675:T26, "Parameters.Properties.Service Channels Status Lookup"=w670:variant, "Service Channels Status"=w667:T26, "Parameters.Properties.Frames Lookup"=w680:variant, "Reads"=w668:T26, "XNETEngine (GMLAN)"=w677:T25, "ADCS Connection"=w672:T19, "Parameters.Properties.CAN.Diagnostic Protocol"=w679:T6)
          n182 = Unbundle By Name(w678) -> ("PID IDs"=w681:u32[])
          n183 = case shown="\"GMLAN\"" w679 {
            tunnel: [w698 w749] -> w674
            tunnel: [w694 _] -> w683
            tunnel: w682 -> [w699 w749]
            tunnel: w681 -> [w696 _]
            tunnel: w680 -> [w691 _]
            tunnel: w672 -> [w697 w748]
            tunnel: [w695 w748] -> w671
            tunnel: w677 -> [w693 _]
            tunnel: [w692 _] -> w673
            tunnel: w668 -> [w690 _]
            tunnel: w667 -> [w689 _]
            tunnel: w670 -> [w688 _]
            frame "GMLAN" {
              n184 = disable-structure shown="InlinePID==FALSE, Default" {
                disable-tunnel: w699 -> [w707 w732]
                disable-tunnel: [w706 w722] -> w698
                disable-tunnel: w697 -> [w705 w731]
                disable-tunnel: w696 -> [w704 w730]
                disable-tunnel: [w703 w729] -> w695
                disable-tunnel: [w702 w728] -> w694
                disable-tunnel: w693 -> [w701 _]
                disable-tunnel: [w700 w727] -> w692
                disable-tunnel: w691 -> [_ w726]
                disable-tunnel: w690 -> [_ w725]
                disable-tunnel: w689 -> [_ w724]
                disable-tunnel: w688 -> [_ w723]
                frame condition #0 {
                  n185 = for {
                    shift-right: [w713] -> w712
                    shift-left: w707 -> [w721]
                    shift-right: [w719] -> w703
                    shift-left: w705 -> [w720]
                    tunnel: w704 -> [w715] mode=indexing
                    tunnel: [w718] -> w702 mode=indexing
                    tunnel: [w717] -> w708 mode=indexing
                    tunnel: [w714] -> w700
                    stop <- w713 stop-if-true
                    n186 = call "GMLAN ReadDataByParameterIdentifier.vi"("error in (no error)"=w721, "Parameter ID (PID)"=w715, "diag ref in"=w720) -> ("error out"=w713:errorcluster, "success?"=w718:bool, "data out"=w714:u8[], "diag ref out"=w719:T19)  [unwired: 5 in]
                    n187 = Bundle By Name(cluster=T36 {"ID"=0, "Raw Frame"=[], "error out"={"status"=FALSE, "code"=0, "source"=""}}, "ID"=w715, "Raw Frame"=w714, "error out"=w713) -> (w717:T36)
                  }
                  n188 = Flatten To String(anything=w708, error in (no error)=w712) -> (data string=w709:string, error out=w711:errorcluster)  [unwired: 2 in, 1 out]
                  n189 = call <vilib>:"Send Local Message.vi"("message queue in"=w701, "message name"="UpdatePIDsOnDemand" ("Message Name"), "message value"=w709, "error in"=w711) -> ("error out"=w706:errorcluster)  [unwired: 9 in, 2 out]
                }
                frame condition #1 (active) {
                  n190 = for {
                    shift-right: [w740] -> w722
                    shift-left: w732 -> [w747]
                    shift-right: [w745] -> w729
                    shift-left: w731 -> [w746]
                    tunnel: w730 -> [w739] mode=indexing
                    tunnel: [w744] -> w728 mode=indexing
                    tunnel: [w738] -> w727
                    tunnel: w726 -> [w737]
                    tunnel: w725 -> [w736]
                    tunnel: w724 -> [w735]
                    tunnel: w723 -> [w734]
                    stop <- w740 stop-if-true
                    w733 = TRUE ("Buffer?")
                    w742 = Type."PID" ("Type")
                    n191 = call "GMLAN ReadDataByParameterIdentifier.vi"("error in (no error)"=w747, "Parameter ID (PID)"=w739, "diag ref in"=w746) -> ("error out"=w741:errorcluster, "success?"=w744:bool, "data out"=w738:u8[], "diag ref out"=w745:T19)  [unwired: 5 in]
                    n192 = call "Signals.Scale.EU.vi"("Buffer?"=w733, "Type"=w742, "Lookup"=w737, "error in (no error)"=w741, "Unscaled Data"=w738, "ID"=w739, "Reads Ref"=w736) -> ("error out"=w743:errorcluster)  [unwired: 4 in]
                    n193 = call "ServiceChannels.Status.Set.vi"("Buffer?"=w733, "Type"=w742, "Status Lookup"=w734, "error in (no error)"=w743, "ID"=w739, "Service Channels Status Ref"=w735) -> ("error out"=w740:errorcluster)  [unwired: 5 in]
                  }
                }
              }
            }
            frame "KWP-2000".."User-Defined" {
            }
          }
          n194 = And Array Elements(Boolean array=w683) -> (logical AND=w676:bool)
          n195 = call "Status.Set.vi"("error in (no error)"=w674, "success?"=w676, "Data"=w673, "Status Ref"=w675) -> ("error out"=w669:errorcluster)  [unwired: 7 in]
          n196 = call-poly <vilib>:"Data.Processes.Execute.vi"("error in (no error)"=w669, "Ref"=w668) -> ("error out"=w666:errorcluster)  [unwired: 9 in]
          n197 = flat-sequence {
            tunnel: w667 -> [w687]
            tunnel: w666 -> [w686]
            tunnel: [w684] -> w665
            frame #0 {
              n198 = call-poly <vilib>:"Data.Processes.Execute.vi"("Ref"=w687) -> ("error out"=w685:errorcluster)  [unwired: 10 in]
              n199 = Merge Errors(w686, w685) -> (w684:errorcluster)
            }
          }
          n200 = in-place-cluster #11("Status"=w675, "Parameters.Properties.Service Channels Status Lookup"=w670, "Service Channels Status"=w667, "Parameters.Properties.Frames Lookup"=w680, "Reads"=w668, "XNETEngine (GMLAN)"=w677, "ADCS Connection"=w671, "Parameters.Properties.CAN.Diagnostic Protocol"=w679) -> (w661:T1)
        }
      }
      frame "ReadPIDOnDemand" {
        n201 = in-place {
          in-place-border: w757 -> [w774]
          in-place-border: w756 -> [w773]
          in-place-border: [w763] -> w755
          in-place-border: w751 -> [_]
          in-place-border: w750 -> [_]
          n202 = in-place-cluster #12(w754) -> ("Status"=w769:T26, "Parameters.Properties.Service Channels Status Lookup"=w758:variant, "Service Channels Status"=w759:T26, "Parameters.Properties.Frames Lookup"=w772:variant, "Reads"=w760:T26, "XNETEngine (GMLAN)"=w770:T25, "ADCS Connection"=w762:T19, "Parameters.Properties.CAN.Diagnostic Protocol"=w771:T6)
          n203 = Unflatten From String(type=u16 0 ("ID"), binary string=w773, error in (no error)=w774) -> (value=w765:u16, error out=w775:errorcluster)  [unwired: 2 in, 1 out]
          n204 = case shown="\"GMLAN\"" w771 {
            tunnel: [w780 w812] -> w768
            tunnel: [w784 _] -> w764
            tunnel: w775 -> [w788 w812]
            tunnel: w765 -> [w786 _]
            tunnel: w772 -> [w779 _]
            tunnel: w762 -> [w787 w811]
            tunnel: [w785 w811] -> w761
            tunnel: w770 -> [w783 _]
            tunnel: [w782 _] -> w767
            tunnel: w760 -> [w778 _]
            tunnel: w759 -> [w777 _]
            tunnel: w758 -> [w776 _]
            frame "GMLAN" {
              n205 = call "GMLAN ReadDataByParameterIdentifier.vi"("error in (no error)"=w788, "Parameter ID (PID)"=w786, "diag ref in"=w787) -> ("error out"=w781:errorcluster, "success?"=w784:bool, "data out"=w782:u8[], "diag ref out"=w785:T19)  [unwired: 5 in]
              n206 = disable-structure shown="InlinePID==FALSE, Default" {
                disable-tunnel: w786 -> [w797 w806]
                disable-tunnel: w783 -> [w796 _]
                disable-tunnel: w782 -> [w795 w805]
                disable-tunnel: w781 -> [w789 w808]
                disable-tunnel: [w791 w807] -> w780
                disable-tunnel: w779 -> [_ w804]
                disable-tunnel: w778 -> [_ w803]
                disable-tunnel: w777 -> [_ w802]
                disable-tunnel: w776 -> [_ w801]
                frame condition #0 {
                  n207 = Bundle By Name(cluster=T36 {"ID"=0, "Raw Frame"=[], "error out"={"status"=FALSE, "code"=0, "source"=""}}, "ID"=w797, "Raw Frame"=w795, "error out"=w789) -> (w798:T36)
                  n208 = Build Array(w798) -> (w790:T36[])
                  n209 = Flatten To String(anything=w790) -> (data string=w793:string, error out=w800:errorcluster)  [unwired: 3 in, 1 out]
                  n210 = call <vilib>:"Send Local Message.vi"("message queue in"=w796, "message name"="UpdatePIDsOnDemand" ("Message Name"), "message value"=w793, "error in"=w800) -> ("error out"=w792:errorcluster)  [unwired: 9 in, 2 out]
                  n211 = Merge Errors(w789, w792) -> (w791:errorcluster)
                }
                frame condition #1 (active) {
                  w809 = Type."PID" ("Type")
                  n212 = call "Signals.Scale.EU.vi"("Type"=w809, "Lookup"=w804, "error in (no error)"=w808, "Unscaled Data"=w805, "ID"=w806, "Reads Ref"=w803) -> ("error out"=w810:errorcluster)  [unwired: 5 in]
                  n213 = call "ServiceChannels.Status.Set.vi"("Type"=w809, "Status Lookup"=w801, "error in (no error)"=w810, "ID"=w806, "Service Channels Status Ref"=w802) -> ("error out"=w807:errorcluster)  [unwired: 6 in]
                }
              }
            }
            frame "KWP-2000".."User-Defined" {
            }
          }
          n214 = call "Status.Set.vi"("error in (no error)"=w768, "success?"=w764, "Data"=w767, "Status Ref"=w769) -> ("error out"=w763:errorcluster)  [unwired: 7 in]
          n215 = in-place-cluster #12("Status"=w769, "Parameters.Properties.Service Channels Status Lookup"=w758, "Service Channels Status"=w759, "Parameters.Properties.Frames Lookup"=w772, "Reads"=w760, "XNETEngine (GMLAN)"=w770, "ADCS Connection"=w761, "Parameters.Properties.CAN.Diagnostic Protocol"=w771) -> (w753:T1)
        }
      }
      frame "StopPIDs" {
        n216 = in-place {
          in-place-border: w816 -> [w827]
          in-place-border: [w826] -> w815
          n217 = in-place-cluster #13(w814) -> ("Status"=w825:T26, "ADCS Connection"=w823:T19, "Parameters.Properties.DPIDs"=w824:T14[], "Parameters.Properties.CAN.Diagnostic Protocol"=w819:T6)
          n218 = case shown="\"GMLAN\"" w819 {
            selector: w819 -> [w828 w833]
            tunnel: w827 -> [w829 w851]
            tunnel: [w829 w849] -> w826
            tunnel: w825 -> [w830 w835]
            tunnel: w824 -> [w832 w834]
            tunnel: w823 -> [w831 w842]
            tunnel: [w831 w839] -> w822
            tunnel: [w830 w835] -> w821
            tunnel: [w832 w834] -> w820
            tunnel: [w828 w833] -> w818
            frame Default {
            }
            frame "GMLAN" {
              w853 = Property_ID."Timeout Diag Command" ("property ID")
              n219 = for {
                tunnel: w834 -> [w868] mode=indexing
                tunnel: [w867] -> w846 mode=indexing
                n220 = Unbundle By Name(w868) -> ("DPID ID"=w867:u8)
              }
              n221 = call <vilib>:"Diag Get Property.vi"("error in (no error)"=w851, "property ID"=w853, "diag ref in"=w842) -> ("error out"=w855:errorcluster, "property value"=w848:u32, "diag ref out"=w843:T19)  [unwired: 6 in]
              n222 = call <vilib>:"Diag Set Property.vi"("error in (no error)"=w855, "property value"=u32 100, "property ID"=w853, "diag ref in"=w843) -> ("error out"=w850:errorcluster, "diag ref out"=w841:T19)  [unwired: 6 in]
              n223 = Empty Array?(array=w846) -> (empty?=w847:bool)
              n224 = case shown="False" w847 {
                tunnel: w850 -> [w863 w865]
                tunnel: [w862 w865] -> w838
                tunnel: w841 -> [w861 w866]
                tunnel: [w860 w866] -> w840
                tunnel: ReadDataByPacketIdentifier_SubFunctions."stopSending" ("Sub Function") -> [w859 _]
                tunnel: w846 -> [w858 _]
                tunnel: [w857 TRUE ("success?")] -> w837
                tunnel: [w856 _] -> w836
                frame False {
                  n225 = call "GMLAN ReadDataByPacketIdentifier.vi"("error in (no error)"=w863, "DPIDs"=w858, "Sub Function"=w859, "diag ref in"=w861) -> ("error out"=w862:errorcluster, "success?"=w857:bool, "data out"=w856:u8[], "diag ref out"=w860:T19)  [unwired: 4 in]
                }
                frame True {
                }
              }
              n226 = call "Status.Set.vi"("error in (no error)"=w838, "success?"=w837, "Data"=w836, "Status Ref"=w835) -> ("error out"=w845:errorcluster)  [unwired: 7 in]
              n227 = call <vilib>:"Diag Set Property.vi"("error in (no error)"=w845, "property value"=w848, "property ID"=Property_ID."Timeout Diag Command", "diag ref in"=w840) -> ("error out"=w849:errorcluster, "diag ref out"=w839:T19)  [unwired: 6 in]
            }
          }
          n228 = in-place-cluster #13("Status"=w821, "ADCS Connection"=w822, "Parameters.Properties.DPIDs"=w820, "Parameters.Properties.CAN.Diagnostic Protocol"=w818) -> (w813:T1)
        }
      }
      frame "GenerateCPID" {
        n229 = in-place {
          in-place-border: w873 -> [w891]
          in-place-border: w872 -> [w890]
          in-place-border: [w884] -> w871
          n230 = in-place-cluster #14(w870) -> ("Status"=w883:T26, "Parameters.Properties.Service Channels Status Lookup"=w878:variant, "Service Channels Status"=w877:T26, "ADCS Connection"=w889:T19, "Parameters.Properties.CAN.Diagnostic Protocol"=w882:T6, "Parameters.Properties.Frames Lookup"=w887:variant, "Writes"=w886:T27)
          n231 = case shown="\"GMLAN\"" w882 {
            selector: w882 -> [w897 w908]
            tunnel: w891 -> [w894 w919]
            tunnel: w890 -> [_ w918]
            tunnel: w889 -> [w898 w917]
            tunnel: [w898 w916] -> w888
            tunnel: w887 -> [w896 w909]
            tunnel: w886 -> [w895 w907]
            tunnel: [w895 w907] -> w885
            tunnel: [w894 w912] -> w884
            tunnel: w883 -> [w899 w910]
            tunnel: [w899 w910] -> w881
            tunnel: [w897 w908] -> w880
            tunnel: [w896 w909] -> w879
            tunnel: w878 -> [w892 w901]
            tunnel: w877 -> [w893 w900]
            tunnel: [w892 w901] -> w876
            tunnel: [w893 w900] -> w875
            frame Default {
            }
            frame "GMLAN" {
              w903 = Type."CPID" ("Type")
              n232 = Unflatten From String(type=u16 0, binary string=w918, error in (no error)=w919) -> (value=w902:u16, error out=w906:errorcluster)  [unwired: 2 in, 1 out]
              n233 = call "Signals.Scale.Raw.vi"("Type"=w903, "Lookup"=w909, "error in"=w906, "ID"=w902, "Writes Ref"=w907) -> ("error out"=w914:errorcluster, "Data"=w913:u8[])  [unwired: 5 in]
              n234 = call "GMLAN DeviceControl.vi"("error in (no error)"=w914, "CPIDControlBytes"=w913, "CPID ID"=w902, "diag ref in"=w917) -> ("error out"=w905:errorcluster, "success?"=w911:bool, "diag ref out"=w916:T19)  [unwired: 5 in]
              n235 = call "ServiceChannels.Status.Set.vi"("Type"=w903, "Status Lookup"=w901, "error in (no error)"=w905, "ID"=w902, "Service Channels Status Ref"=w900) -> ("error out"=w904:errorcluster)  [unwired: 6 in]
              n236 = call "Status.Set.vi"("error in (no error)"=w904, "success?"=w911, "Status Ref"=w910) -> ("error out"=w912:errorcluster)  [unwired: 8 in]
            }
          }
          n237 = in-place-cluster #14("Status"=w881, "Parameters.Properties.Service Channels Status Lookup"=w876, "Service Channels Status"=w875, "ADCS Connection"=w888, "Parameters.Properties.CAN.Diagnostic Protocol"=w880, "Parameters.Properties.Frames Lookup"=w879, "Writes"=w885) -> (w869:T1)
        }
      }
      frame "<--------------- GENERIC SERVICES --------------->" {
      }
      frame "StopCANComm" {
        # "Stopping so don't need to send a tester present message."
        n238 = in-place {
          in-place-border: [w932] -> w928
          n239 = in-place-dvr #15(w930) -> (w932:errorcluster)  [unwired: 1 out]
          n240 = in-place-dvr #15(TRUE ("data value")) -> (w929:errorcluster)  [unwired: 1 out]
        }
        n241 = Merge Errors(w927, w929, w928) -> (w926:errorcluster)
        n242 = Bundle By Name(cluster=w924, "TesterPresentEnabled?"=FALSE) -> (w923:T31)
      }
      frame "DisableRepeatingTesterPresent" {
        n243 = Bundle By Name(cluster=w936, "TesterPresentEnabled?"=FALSE) -> (w935:T31)
      }
      frame "EnableRepeatingTesterPresent" {
        n244 = Bundle By Name(cluster=w940, "TesterPresentEnabled?"=TRUE) -> (w939:T31)
      }
      frame "ForceTesterPresent" {
        n245 = in-place {
          in-place-border: w948 -> [w958]
          in-place-border: [w953] -> w947
          in-place-border: w944 -> [w955]
          n246 = in-place-cluster #16(w946) -> ("Status"=w952:T26, "Parameters.Properties.CAN.Diagnostic Protocol"=w960:T6, "ADCS Connection"=w962:T19)
          n247 = Unflatten From String(type=FALSE, binary string=w955, error in (no error)=w958) -> (value=w956:bool, error out=w957:errorcluster)  [unwired: 2 in, 1 out]
          n248 = case shown="\"KWP-2000\"" w960 {
            tunnel: w957 -> [w964 w971 w974 w981]
            tunnel: [w963 w971 w973 w983] -> w954
            tunnel: w962 -> [w968 w969 w980 w986]
            tunnel: [w967 w969 w979 w985] -> w961
            tunnel: w956 -> [w966 _ w976 w984]
            tunnel: [w965 FALSE ("success?") w972 w982] -> w951
            frame "KWP-2000" {
              n249 = call <vilib>:"TesterPresent.vi"("error in (no error)"=w964, "response required?"=w966, "diag ref in"=w968) -> ("error out"=w963:errorcluster, "success?"=w965:bool, "diag ref out"=w967:T19)  [unwired: 6 in]
            }
            frame "User-Defined" {
            }
            frame "GMLAN" {
              n250 = Select(t=TesterPresent_Parameter."SpecificECU" ("Parameter"), s=w976, f=TesterPresent_Parameter."EntireNetwork" ("Parameter")) -> (s? t:f=w975:T38)
              n251 = call "GMLAN TesterPresent.vi"("error in (no error)"=w974, "Parameter"=w975, "diag ref in"=w980) -> ("error out"=w973:errorcluster, "success?"=w972:bool, "diag ref out"=w979:T19)  [unwired: 6 in]
            }
            frame "UDS" {
              n252 = call <vilib>:"UDS TesterPresent.vi"("error in (no error)"=w981, "response required?"=w984, "diag ref in"=w986) -> ("error out"=w983:errorcluster, "success?"=w982:bool, "diag ref out"=w985:T19)  [unwired: 6 in]
            }
          }
          n253 = call "Status.Set.vi"("error in (no error)"=w954, "success?"=w951, "Status Ref"=w952) -> ("error out"=w953:errorcluster)  [unwired: 8 in]
          n254 = in-place-cluster #16("Status"=w952, "Parameters.Properties.CAN.Diagnostic Protocol"=w960, "ADCS Connection"=w961) -> (w945:T1)
        }
      }
      frame "ClearSuccessBit" {
        n255 = in-place {
          in-place-border: w990 -> [w994]
          in-place-border: [w992] -> w989
          n256 = in-place-cluster #17(w988) -> ("Status"=w995:T26)
          n257 = call "Status.Set.vi"("error in (no error)"=w994, "success?"=FALSE ("Boolean"), "Status Ref"=w995) -> ("error out"=w992:errorcluster)  [unwired: 8 in]
          n258 = in-place-cluster #17("Status"=w995) -> (w987:T1)
        }
      }
      frame "EnableDiagnosticSession" {
        n259 = in-place {
          in-place-border: w1000 -> [w1010]
          in-place-border: [w1003] -> w999
          in-place-border: w998 -> [w1009]
          n260 = in-place-cluster #18(w997) -> ("Status"=w1002:T26, "Parameters.Properties.CAN.Diagnostic Protocol"=w1006:T6, "ADCS Connection"=w1008:T19)
          n261 = Unflatten From String(type=u8 0 ("ID"), binary string=w1009, error in (no error)=w1010) -> (value=w1012:u8, error out=w1011:errorcluster)  [unwired: 2 in, 1 out]
          n262 = case shown="\"User-Defined\"" w1006 {
            tunnel: [w1017 w1023 w1029 w1032] -> w1005
            tunnel: [w1019 FALSE ("success?") w1028 w1031] -> w1004
            tunnel: w1012 -> [w1014 _ w1027 w1034]
            tunnel: w1011 -> [w1018 w1023 w1026 w1033]
            tunnel: w1008 -> [w1016 w1022 w1025 w1035]
            tunnel: [w1015 w1022 w1024 w1030] -> w1007
            frame "GMLAN" {
              n263 = call "GMLAN InitiateDiagnosticOperation.vi"("error in (no error)"=w1018, "SubFunctions"=w1014, "Parameter"=InitiateDiagnosticOperation_Parameter."SpecificECU", "diag ref in"=w1016) -> ("error out"=w1017:errorcluster, "success?"=w1019:bool, "diag ref out"=w1015:T19)  [unwired: 5 in]
            }
            frame "User-Defined" {
            }
            frame "UDS" {
              n264 = call <vilib>:"UDS DiagnosticSessionControl.vi"("error in (no error)"=w1026, "mode"=w1027, "diag ref in"=w1025) -> ("error out"=w1029:errorcluster, "success?"=w1028:bool, "diag ref out"=w1024:T19)  [unwired: 5 in, 1 out]
            }
            frame "KWP-2000" {
              n265 = call <vilib>:"StartDiagnosticSession.vi"("error in (no error)"=w1033, "mode"=w1034, "diag ref in"=w1035) -> ("error out"=w1032:errorcluster, "success?"=w1031:bool, "diag ref out"=w1030:T19)  [unwired: 6 in]
            }
          }
          n266 = call "Status.Set.vi"("error in (no error)"=w1005, "success?"=w1004, "Status Ref"=w1002) -> ("error out"=w1003:errorcluster)  [unwired: 8 in]
          n267 = in-place-cluster #18("Status"=w1002, "Parameters.Properties.CAN.Diagnostic Protocol"=w1006, "ADCS Connection"=w1007) -> (w996:T1)
        }
      }
      frame "DisableDiagnosticSession" {
        n268 = in-place {
          in-place-border: [w1042] -> w1039
          in-place-border: w1038 -> [w1048]
          n269 = in-place-cluster #19(w1037) -> ("Status"=w1041:T26, "Parameters.Properties.CAN.Diagnostic Protocol"=w1045:T6, "ADCS Connection"=w1047:T19)
          n270 = case shown="\"User-Defined\"" w1045 {
            tunnel: [w1051 w1057 w1060 w1069] -> w1044
            tunnel: [w1053 FALSE ("success?") w1059 w1068] -> w1043
            tunnel: w1048 -> [w1050 w1057 w1063 w1066]
            tunnel: w1047 -> [w1049 w1058 w1062 w1065]
            tunnel: [w1052 w1058 w1061 w1064] -> w1046
            frame "GMLAN" {
              w1054 = T53 2 items=["disableAllDTCs"=2, "enableDTCsDuringDevCntrl"=3, "wakeUpLinks"=4] ("SubFunctions")
              n271 = call "GMLAN InitiateDiagnosticOperation.vi"("error in (no error)"=w1050, "SubFunctions"=w1054, "Parameter"=InitiateDiagnosticOperation_Parameter."SpecificECU", "diag ref in"=w1049) -> ("error out"=w1051:errorcluster, "success?"=w1053:bool, "diag ref out"=w1052:T19)  [unwired: 5 in]
            }
            frame "User-Defined" {
            }
            frame "KWP-2000" {
              n272 = call <vilib>:"StopDiagnosticSession.vi"("error in (no error)"=w1063, "diag ref in"=w1062) -> ("error out"=w1060:errorcluster, "success?"=w1059:bool, "diag ref out"=w1061:T19)  [unwired: 7 in]
            }
            frame "UDS" {
              n273 = call <vilib>:"UDS DiagnosticSessionControl.vi"("error in (no error)"=w1066, "mode"=u8 1, "diag ref in"=w1065) -> ("error out"=w1069:errorcluster, "success?"=w1068:bool, "diag ref out"=w1064:T19)  [unwired: 5 in, 1 out]
            }
          }
          n274 = call "Status.Set.vi"("error in (no error)"=w1044, "success?"=w1043, "Status Ref"=w1041) -> ("error out"=w1042:errorcluster)  [unwired: 8 in]
          n275 = in-place-cluster #19("Status"=w1041, "Parameters.Properties.CAN.Diagnostic Protocol"=w1045, "ADCS Connection"=w1046) -> (w1036:T1)
        }
      }
      frame "DisableNormalCommunication" {
        n276 = in-place {
          in-place-border: [w1083] -> w1074
          in-place-border: w1073 -> [w1081]
          in-place-border: w1070 -> [w1079]
          n277 = in-place-cluster #20(w1072) -> ("Status"=w1086:T26, "Parameters.Properties.CAN.Diagnostic Protocol"=w1087:T6, "ADCS Connection"=w1089:T19)
          n278 = Unflatten From String(type=T40 {"Type"=0, "CommType"=0} ("Cluster"), binary string=w1079, error in (no error)=w1081) -> (value=w1082:T40, error out=w1080:errorcluster)  [unwired: 2 in, 1 out]
          n279 = Unbundle By Name(w1082) -> ("Type"=w1077:u8, "CommType"=w1076:u8)
          n280 = case shown="\"User-Defined\"" w1087 {
            tunnel: w1089 -> [w1095 w1101 w1109 w1114]
            tunnel: [w1096 w1101 w1108 w1113] -> w1088
            tunnel: [w1098 w1102 w1107 w1111] -> w1084
            tunnel: [w1097 FALSE ("success?") w1106 w1112] -> w1085
            tunnel: w1080 -> [w1099 w1102 w1105 w1115]
            tunnel: w1077 -> [w1094 _ w1104 _]
            tunnel: w1076 -> [_ _ w1103 _]
            frame "GMLAN" {
              n281 = Not Equal To 0?(x=w1094) -> (x != 0?=w1093:bool)
              n282 = Select(t=DisableNormalCommunication_Parameter."SpecificECU" ("Parameter"), s=w1093, f=DisableNormalCommunication_Parameter."EntireNetwork" ("Parameter")) -> (s? t:f=w1091:T41)
              n283 = call "GMLAN DisableNormalCommunication.vi"("error in (no error)"=w1099, "Parameter"=w1091, "diag ref in"=w1095) -> ("error out"=w1098:errorcluster, "success?"=w1097:bool, "diag ref out"=w1096:T19)  [unwired: 6 in]
            }
            frame "User-Defined" {
            }
            frame "UDS" {
              n284 = call <vilib>:"UDS CommunicationControl.vi"("error in (no error)"=w1105, "communication type"=w1103, "type"=w1104, "diag ref in"=w1109) -> ("error out"=w1107:errorcluster, "success?"=w1106:bool, "diag ref out"=w1108:T19)  [unwired: 5 in]
            }
            frame "KWP-2000" {
              n285 = call <vilib>:"DisableNormalMessageTransmission.vi"("error in (no error)"=w1115, "require response?"=TRUE, "diag ref in"=w1114) -> ("error out"=w1111:errorcluster, "success?"=w1112:bool, "diag ref out"=w1113:T19)  [unwired: 6 in]
            }
          }
          n286 = call "Status.Set.vi"("error in (no error)"=w1084, "success?"=w1085, "Status Ref"=w1086) -> ("error out"=w1083:errorcluster)  [unwired: 8 in]
          n287 = in-place-cluster #20("Status"=w1086, "Parameters.Properties.CAN.Diagnostic Protocol"=w1087, "ADCS Connection"=w1088) -> (w1071:T1)
        }
      }
      frame "ReturnToNormalMode" {
        n288 = in-place {
          in-place-border: [w1122] -> w1119
          in-place-border: w1118 -> [w1128]
          n289 = in-place-cluster #21(w1117) -> ("Status"=w1121:T26, "ADCS Connection"=w1127:T19, "Parameters.Properties.CAN.Diagnostic Protocol"=w1125:T6)
          n290 = case shown="\"GMLAN\"" w1125 {
            tunnel: [w1131 w1136 w1143 w1145] -> w1124
            tunnel: [w1129 FALSE ("success?") w1142 w1146] -> w1123
            tunnel: w1128 -> [w1133 w1136 w1139 w1149]
            tunnel: w1127 -> [w1132 w1135 w1138 w1148]
            tunnel: [w1130 w1135 w1137 w1147] -> w1126
            frame "GMLAN" {
              n291 = call "GMLAN ReturnToNormalMode.vi"("error in (no error)"=w1133, "diag ref in"=w1132) -> ("error out"=w1131:errorcluster, "success?"=w1129:bool, "diag ref out"=w1130:T19)  [unwired: 7 in]
            }
            frame "User-Defined" {
            }
            frame "UDS" {
              n292 = call <vilib>:"UDS CommunicationControl.vi"("error in (no error)"=w1139, "communication type"=u8 3 ("type"), "type"=u8 0, "diag ref in"=w1138) -> ("error out"=w1143:errorcluster, "success?"=w1142:bool, "diag ref out"=w1137:T19)  [unwired: 5 in]
            }
            frame "KWP-2000" {
              n293 = call <vilib>:"EnableNormalMessageTransmission.vi"("error in (no error)"=w1149, "require response?"=TRUE, "diag ref in"=w1148) -> ("error out"=w1145:errorcluster, "success?"=w1146:bool, "diag ref out"=w1147:T19)  [unwired: 6 in]
            }
          }
          n294 = call "Status.Set.vi"("error in (no error)"=w1124, "success?"=w1123, "Status Ref"=w1121) -> ("error out"=w1122:errorcluster)  [unwired: 8 in]
          n295 = in-place-cluster #21("Status"=w1121, "ADCS Connection"=w1126, "Parameters.Properties.CAN.Diagnostic Protocol"=w1125) -> (w1116:T1)
        }
      }
      frame "UnlockECU" {
        n296 = in-place {
          in-place-border: w1153 -> [w1163]
          in-place-border: [w1159] -> w1152
          n297 = in-place-cluster #22(w1151) -> ("Status"=w1157:T26, "ADCS Connection"=w1162:T19, "Parameters.Properties.CAN.Security"=w1155:T8, "Parameters.Properties.CAN.Diagnostic Protocol"=w1156:T6)
          n298 = case shown="\"GMLAN\"..\"UDS\"" w1156 {
            selector: w1156 -> [_ w1167]
            tunnel: w1163 -> [w1166 w1173]
            tunnel: w1162 -> [w1164 w1172]
            tunnel: w1155 -> [_ w1171]
            tunnel: [w1164 w1170] -> w1161
            tunnel: [w1166 w1169] -> w1160
            tunnel: [FALSE ("success?") w1168] -> w1158
            frame "User-Defined" {
            }
            frame "GMLAN".."UDS" {
              n299 = call "ADCS.UnlockECUSecurity.vi"("Diagnostic Protocol"=w1167, "error in (no error)"=w1173, "Security"=w1171, "diag ref in"=w1172) -> ("error out"=w1169:errorcluster, "success?"=w1168:bool, "diag ref out"=w1170:T19)  [unwired: 5 in]
            }
          }
          n300 = call "Status.Set.vi"("error in (no error)"=w1160, "success?"=w1158, "Status Ref"=w1157) -> ("error out"=w1159:errorcluster)  [unwired: 8 in]
          n301 = in-place-cluster #22("Status"=w1157, "ADCS Connection"=w1161, "Parameters.Properties.CAN.Security"=w1155, "Parameters.Properties.CAN.Diagnostic Protocol"=w1156) -> (w1150:T1)
        }
      }
      frame "ReadDTCs" {
        n302 = in-place {
          in-place-border: [w1203] -> w1183
          in-place-border: w1182 -> [w1202]
          in-place-border: w1181 -> [w1201]
          in-place-border: w1180 -> [w1200]
          in-place-border: w1179 -> [w1199]
          in-place-border: w1174 -> [w1184]
          n303 = in-place-cluster #23(w1178) -> ("Status"=w1195:T26, "DTC Count"=w1192:T26, "DTCs"=w1191:T26, "Parameters.Properties.DTC.Descriptor"=w1194:T17, "ADCS Connection"=w1197:T19, "Parameters.Properties.CAN.Diagnostic Protocol"=w1190:T6)
          n304 = in-place-cluster #24(w1177) -> ("Active DTCs"=w1198:T30[])
          n305 = case shown="\"KWP-2000\", \"UDS\"" w1190 {
            selector: w1190 -> [w1216 w1219 w1244]
            tunnel: [w1212 w1217 w1254] -> w1203
            tunnel: w1202 -> [w1205 _ w1231]
            tunnel: w1201 -> [w1213 w1217 w1253]
            tunnel: w1200 -> [_ _ w1252]
            tunnel: w1199 -> [_ _ w1251]
            tunnel: w1198 -> [w1211 w1218 w1248]
            tunnel: w1197 -> [w1210 w1220 w1247]
            tunnel: [w1211 w1218 w1246] -> w1196
            tunnel: w1195 -> [w1206 w1224 w1240]
            tunnel: w1194 -> [w1209 w1221 w1226]
            tunnel: [w1210 w1220 w1245] -> w1193
            tunnel: w1192 -> [w1207 w1223 w1242]
            tunnel: w1191 -> [w1208 w1222 w1243]
            tunnel: [w1216 w1219 w1244] -> w1189
            tunnel: [w1209 w1221 w1226] -> w1188
            tunnel: [w1208 w1222 w1243] -> w1187
            tunnel: [w1207 w1223 w1242] -> w1186
            tunnel: [w1206 w1224 w1240] -> w1185
            tunnel: w1184 -> [w1204 _ w1230]
            frame "GMLAN" {
              n306 = Flatten To String(anything=w1211, error in (no error)=w1213) -> (data string=w1214:string, error out=w1215:errorcluster)  [unwired: 2 in, 1 out]
              n307 = call <vilib>:"Respond to Command.vi"("error in (no error)"=w1215, "message value"=w1214, "ResponseInfo"=w1205, "VeriStand Comm in"=w1204) -> ("error out"=w1212:errorcluster)  [unwired: 5 in, 2 out]
            }
            frame "User-Defined" {
            }
            frame "KWP-2000", "UDS" {
              n308 = Unflatten From String(type=T42 {"Extension"=0, "Mask"=0, "Mode"=0, "Byte Lengths"={"Override"=FALSE, "DTC"=0, "Status"=0, "Failure"=0}}, binary string=w1252, error in (no error)=w1253) -> (value=w1228:T42, error out=w1250:errorcluster)  [unwired: 2 in, 1 out]
              n309 = Unbundle By Name(w1228) -> ("Byte Lengths"=w1227:T43)
              n310 = Unbundle By Name(w1228) -> ("Extension"=w1236:u32, "Mode"=w1235:u32, "Mask"=w1234:u32)
              n311 = call "DTC.Descriptor.Override.vi"("Byte Lengths"=w1227, "Descriptor in"=w1226) -> ("Descriptor out"=w1225:T17)  [unwired: 9 in]
              n312 = case shown="\"UDS\"" w1244 {
                tunnel: w1225 -> [w1264 w1299 _]
                tunnel: w1250 -> [w1259 w1294 w1317]
                tunnel: w1247 -> [w1258 w1293 w1318]
                tunnel: [w1260 w1295 _] -> w1239
                tunnel: [w1263 w1296 w1317] -> w1241
                tunnel: [w1262 w1298 w1318] -> w1245
                tunnel: [w1261 w1297 _] -> w1249
                tunnel: w1236 -> [w1257 w1292 _]
                tunnel: w1234 -> [w1256 w1291 _]
                tunnel: w1235 -> [w1255 w1290 _]
                frame "UDS" {
                  n313 = case shown="2, Default" w1257 {
                    tunnel: w1264 -> [w1268 w1275 w1289]
                    tunnel: w1256 -> [w1266 w1274 w1288]
                    tunnel: [w1272 w1280 w1287] -> w1263
                    tunnel: [w1269 w1277 w1286] -> w1262
                    tunnel: [w1270 w1278 w1285] -> w1261
                    tunnel: [w1271 w1279 w1284] -> w1260
                    tunnel: w1259 -> [w1273 w1281 w1283]
                    tunnel: w1258 -> [w1267 w1276 w1282]
                    tunnel: w1255 -> [w1265 _ _]
                    frame 8 {
                      n314 = call <vilib>:"UDS ReportDTCBySeverityMaskRecord.vi"("DTC descriptor"=w1268, "error in (no error)"=w1273, "status"=w1266, "severity mask"=w1265, "diag ref in"=w1267) -> ("error out"=w1272:errorcluster, "success?"=w1271:bool, "DTCs"=w1270:T54[], "diag ref out"=w1269:T19)  [unwired: 2 in, 1 out]
                    }
                    frame 9 {
                      n315 = call <vilib>:"UDS ReportSeverityInformationOfDTC.vi"("DTC descriptor"=w1275, "error in (no error)"=w1281, "DTC mask record"=w1274, "diag ref in"=w1276) -> ("error out"=w1280:errorcluster, "success?"=w1279:bool, "DTCs"=w1278:T54[], "diag ref out"=w1277:T19)  [unwired: 3 in, 1 out]
                    }
                    frame 2, Default {
                      n316 = call <vilib>:"UDS ReportDTCByStatusMask.vi"("DTC descriptor"=w1289, "error in (no error)"=w1283, "status mask"=w1288, "diag ref in"=w1282) -> ("error out"=w1287:errorcluster, "success?"=w1284:bool, "DTCs"=w1285:T54[], "diag ref out"=w1286:T19)  [unwired: 3 in, 1 out]
                    }
                  }
                }
                frame "KWP-2000" {
                  n317 = case shown="17, Default" w1292 {
                    tunnel: w1291 -> [w1307 w1316]
                    tunnel: w1299 -> [w1306 w1315]
                    tunnel: [w1305 w1314] -> w1298
                    tunnel: [w1304 w1313] -> w1297
                    tunnel: [w1303 w1312] -> w1296
                    tunnel: [w1302 w1311] -> w1295
                    tunnel: w1294 -> [w1301 w1310]
                    tunnel: w1293 -> [w1300 w1309]
                    tunnel: w1290 -> [_ w1308]
                    frame 23, Default {
                      n318 = call <vilib>:"ReadStatusOfDTC.vi"("DTC descriptor"=w1306, "error in (no error)"=w1301, "group of DTC"=w1307, "diag ref in"=w1300) -> ("error out"=w1303:errorcluster, "success?"=w1302:bool, "DTCs"=w1304:T54[], "diag ref out"=w1305:T19)  [unwired: 4 in]
                    }
                    frame 24 {
                      n319 = call <vilib>:"ReadDTCByStatus.vi"("DTC descriptor"=w1315, "error in (no error)"=w1310, "group of DTC"=w1316, "mode"=w1308, "diag ref in"=w1309) -> ("error out"=w1312:errorcluster, "success?"=w1311:bool, "DTCs"=w1313:T54[], "diag ref out"=w1314:T19)  [unwired: 3 in]
                    }
                  }
                }
                frame "GMLAN", "User-Defined" {
                }
              }
              n320 = case shown="No Error" w1241 {
                selector: w1241 -> [w1320 w1338]
                tunnel: w1243 -> [w1322 _]
                tunnel: w1251 -> [w1330 _]
                tunnel: [w1319 w1338] -> w1238
                tunnel: w1242 -> [w1323 _]
                tunnel: w1249 -> [w1329 _]
                tunnel: w1248 -> [w1328 w1337]
                tunnel: [w1327 w1337] -> w1246
                frame No Error {
                  n321 = Get Date/Time In Seconds() -> (seconds since 1Jan1904=w1326:timestamp)
                  n322 = call "DTCs.List.Update.vi"("current time"=w1326, "Previous Changed DTCs"=w1328, "current DTCs"=w1329) -> ("Active DTCs"=w1327:T30[])  [unwired: 8 in]
                  n323 = Replace Array Subset(array=w1330, new element=w1327, index=0) -> (w1332:T30[])
                  n324 = Array Size(array=w1327) -> (size(s)=w1333:i32)
                  n325 = for {
                    tunnel: w1332 -> [w1336] mode=indexing
                    tunnel: [w1335] -> w1325 mode=concatenating
                    # "Put 10 newest DTCs in VS"
                    n326 = Cluster To Array(cluster=w1336) -> (array=w1335:dbl[])
                  }
                  n327 = To Double Precision Float(number=w1333) -> (double precision float=w1334:dbl)
                  n328 = Build Array(w1334) -> (w1324:dbl[])
                  n329 = call-poly <vilib>:"Data.Processes.Execute.vi"("error in (no error)"=w1320, "Values"=w1324, "Ref"=w1323) -> ("error out"=w1321:errorcluster)  [unwired: 8 in]
                  n330 = call-poly <vilib>:"Data.Processes.Execute.vi"("error in (no error)"=w1321, "Values"=w1325, "Ref"=w1322) -> ("error out"=w1319:errorcluster)  [unwired: 8 in]
                }
                frame Error {
                }
              }
              n331 = call "Status.Set.vi"("error in (no error)"=w1238, "success?"=w1239, "Status Ref"=w1240) -> ("error out"=w1237:errorcluster)  [unwired: 8 in]
              n332 = Flatten To String(anything=w1246, error in (no error)=w1237) -> (data string=w1232:string, error out=w1233:errorcluster)  [unwired: 2 in, 1 out]
              n333 = call <vilib>:"Respond to Command.vi"("error in (no error)"=w1233, "message value"=w1232, "ResponseInfo"=w1231, "VeriStand Comm in"=w1230) -> ("error out"=w1254:errorcluster)  [unwired: 5 in, 2 out]
            }
          }
          n334 = in-place-cluster #23("Status"=w1185, "DTC Count"=w1186, "DTCs"=w1187, "Parameters.Properties.DTC.Descriptor"=w1188, "ADCS Connection"=w1193, "Parameters.Properties.CAN.Diagnostic Protocol"=w1189) -> (w1175:T1)
          n335 = in-place-cluster #24("Active DTCs"=w1196) -> (w1176:T31)
        }
      }
      frame "ClearDTCs" {
        n336 = in-place {
          in-place-border: w1351 -> [w1374]
          in-place-border: w1350 -> [w1373]
          in-place-border: [w1357] -> w1349
          in-place-border: w1348 -> [w1372]
          in-place-border: w1347 -> [w1371]
          in-place-border: w1340 -> [w1354]
          in-place-border: w1339 -> [w1352]
          n337 = in-place-cluster #25(w1346) -> ("Status"=w1359:T26, "DTC Count"=w1366:T26, "DTCs"=w1367:T26, "Parameters.Properties.DTC.Descriptor"=w1368:T17, "Parameters.Properties.CAN.Diagnostic Protocol"=w1363:T6, "ADCS Connection"=w1370:T19, "XNETEngine (GMLAN)"=w1361:T25)
          n338 = case shown="\"KWP-2000\", \"UDS\"" w1363 {
            selector: w1363 -> [w1389 w1397 w1413]
            tunnel: w1374 -> [w1378 _ w1408]
            tunnel: w1373 -> [_ _ _]
            tunnel: [w1383 FALSE ("success?") w1425] -> w1355
            tunnel: [w1375 w1394 w1422] -> w1358
            tunnel: w1372 -> [_ _ w1421]
            tunnel: w1371 -> [w1388 w1394 w1420]
            tunnel: w1370 -> [w1386 w1396 w1417]
            tunnel: [w1385 w1396 w1416] -> w1369
            tunnel: w1368 -> [w1380 w1392 w1402]
            tunnel: w1367 -> [w1391 w1398 w1414]
            tunnel: w1366 -> [w1390 w1399 w1415]
            tunnel: [w1390 w1399 w1415] -> w1365
            tunnel: [w1391 w1398 w1414] -> w1364
            tunnel: [w1389 w1397 w1413] -> w1362
            tunnel: w1361 -> [w1382 w1395 w1412]
            tunnel: [w1382 w1395 w1412] -> w1360
            tunnel: [w1381 w1400 w1411] -> w1356
            tunnel: w1359 -> [w1381 w1400 w1411]
            tunnel: w1354 -> [_ _ w1410]
            tunnel: [w1380 w1392 w1402] -> w1353
            tunnel: w1352 -> [w1377 _ w1407]
            frame "GMLAN" {
              n339 = call <vilib>:"Send Local Message.vi"("message queue in"=w1382, "message name"="ClearDTCs" ("Message Name"), "error in"=w1388) -> ("error out"=w1387:errorcluster)  [unwired: 10 in, 2 out]
              n340 = call "GMLAN ClearDiagnosticInformation.vi"("error in (no error)"=w1387, "diag ref in"=w1386) -> ("error out"=w1376:errorcluster, "success?"=w1383:bool, "diag ref out"=w1385:T19)  [unwired: 7 in]
              n341 = call <vilib>:"Respond to Command.vi"("error in (no error)"=w1376, "message value"="Cleared" ("Message Value"), "ResponseInfo"=w1378, "VeriStand Comm in"=w1377) -> ("error out"=w1375:errorcluster)  [unwired: 5 in, 2 out]
            }
            frame "User-Defined" {
            }
            frame "KWP-2000", "UDS" {
              (unwired) u32 16777215 items=["All"=16777215] ("Group of DTC")
              n342 = Unflatten From String(type=T44 {"Group of DTC"=16777215, "Byte Lengths"={"Override"=FALSE, "DTC"=0, "Status"=0, "Failure"=0}} ("Clear DTC Settings"), binary string=w1421, error in (no error)=w1420) -> (value=w1418:T44, error out=w1419:errorcluster)  [unwired: 2 in, 1 out]
              n343 = Unbundle By Name(w1418) -> ("Byte Lengths"=w1403:T43, "Group of DTC"=w1404:u32)
              n344 = call "DTC.Descriptor.Override.vi"("Byte Lengths"=w1403, "Descriptor in"=w1402) -> ("Descriptor out"=w1401:T17)  [unwired: 9 in]
              n345 = case shown="\"KWP-2000\"" w1413 {
                tunnel: w1417 -> [w1428 w1433 w1442]
                tunnel: [w1428 w1432 w1441] -> w1416
                tunnel: [w1427 w1430 w1440] -> w1406
                tunnel: [FALSE ("success?") w1431 w1439] -> w1425
                tunnel: w1401 -> [_ w1429 w1438]
                tunnel: w1419 -> [w1427 w1435 w1437]
                tunnel: w1404 -> [_ w1434 w1436]
                frame "GMLAN", "User-Defined" {
                }
                frame "KWP-2000" {
                  n346 = call <vilib>:"ClearDiagnosticInformation.vi"("DTC descriptor"=w1429, "error in (no error)"=w1435, "group of DTC"=w1434, "diag ref in"=w1433) -> ("error out"=w1430:errorcluster, "success?"=w1431:bool, "diag ref out"=w1432:T19)  [unwired: 5 in]
                }
                frame "UDS" {
                  n347 = call <vilib>:"UDS ClearDiagnosticInformation.vi"("DTC descriptor"=w1438, "error in (no error)"=w1437, "group of DTC"=w1436, "diag ref in"=w1442) -> ("error out"=w1440:errorcluster, "success?"=w1439:bool, "diag ref out"=w1441:T19)  [unwired: 5 in]
                }
              }
              n348 = call <vilib>:"Respond to Command.vi"("error in (no error)"=w1406, "message value"="Cleared" ("Message Value"), "ResponseInfo"=w1408, "VeriStand Comm in"=w1407) -> ()  [unwired: 5 in, 3 out]
              n349 = call-poly <vilib>:"Data.Processes.Execute.vi"("error in (no error)"=w1406, "Values"=w1410, "Ref"=w1414) -> ("error out"=w1423:errorcluster)  [unwired: 8 in]
              n350 = call-poly <vilib>:"Data.Processes.Execute.vi"("error in (no error)"=w1423, "Values"=dbl[] [0.0] ("element"), "Ref"=w1415) -> ("error out"=w1422:errorcluster)  [unwired: 8 in]
            }
          }
          n351 = call "Status.Set.vi"("error in (no error)"=w1358, "success?"=w1355, "Status Ref"=w1356) -> ("error out"=w1357:errorcluster)  [unwired: 8 in]
          n352 = in-place-cluster #25("Status"=w1356, "DTC Count"=w1365, "DTCs"=w1364, "Parameters.Properties.DTC.Descriptor"=w1353, "Parameters.Properties.CAN.Diagnostic Protocol"=w1362, "ADCS Connection"=w1369, "XNETEngine (GMLAN)"=w1360) -> (w1345:T1)
        }
        n353 = Bundle By Name(cluster=w1344, "Active DTCs"=T30[] [], "status mask"=u8 0) -> (w1341:T31)
      }
      frame "PollDIDs" {
        n354 = in-place {
          in-place-border: w1450 -> [w1464]
          in-place-border: [w1451] -> w1449
          in-place-border: w1446 -> [w1462]
          in-place-border: w1445 -> [w1461]
          n355 = in-place-cluster #26(w1443) -> ("Polling.Queued"=w1458:bool[])
          n356 = in-place-cluster #27(w1448) -> ("Status"=w1469:T26, "Parameters.Properties.Service Channels Status Lookup"=w1453:variant, "Service Channels Status"=w1454:T26, "Reads"=w1466:T26, "ADCS Connection"=w1474:T19, "Parameters.Properties.Frames Lookup"=w1475:variant, "Parameters.Properties.CAN.Diagnostic Protocol"=w1472:T6)
          n357 = Unflatten From String(type=u32 0 ("ID"), binary string=w1462, error in (no error)=w1464) -> (value=w1457:u32, error out=w1463:errorcluster)  [unwired: 2 in, 1 out]
          n358 = Replace Array Subset(array=w1458, new element=FALSE ("new element/subarray"), index=w1457) -> (w1455:bool[])
          n359 = Index Array(array=w1461, index=w1457) -> (element=w1460:T18)
          n360 = Unbundle By Name(w1460) -> ("DID IDs"=w1459:u32[])
          n361 = for {
            shift-right: [w1486] -> w1471
            shift-left: w1463 -> [w1496]
            shift-right: [w1491] -> w1473
            shift-left: w1474 -> [w1493]
            tunnel: w1475 -> [w1492]
            tunnel: w1459 -> [w1484] mode=indexing
            tunnel: [w1495] -> w1476 mode=indexing
            tunnel: w1472 -> [w1494]
            tunnel: [w1490] -> w1467
            tunnel: w1466 -> [w1488]
            tunnel: w1454 -> [w1483]
            tunnel: w1453 -> [w1482]
            stop <- w1486 stop-if-true
            w1481 = TRUE ("Buffer?")
            w1485 = Type."DID" ("Type")
            n362 = case shown="\"GMLAN\", Default" w1494 {
              tunnel: w1496 -> [w1500 w1508 w1513 w1520]
              tunnel: w1493 -> [w1502 w1510 w1512 w1519]
              tunnel: [w1498 w1507 w1513 w1518] -> w1489
              tunnel: [w1503 w1506 FALSE ("success?") w1517] -> w1495
              tunnel: [w1497 w1505 _ w1516] -> w1490
              tunnel: w1484 -> [w1499 w1509 _ w1515]
              tunnel: [w1501 w1504 w1512 w1514] -> w1491
              frame "GMLAN", Default {
                n363 = call "GMLAN ReadDataByIdentifier.vi"("error in (no error)"=w1500, "Data ID (DID)"=w1499, "diag ref in"=w1502) -> ("error out"=w1498:errorcluster, "success?"=w1503:bool, "data out"=w1497:u8[], "diag ref out"=w1501:T19)  [unwired: 5 in]
              }
              frame "KWP-2000" {
                n364 = call <vilib>:"ReadDataByLocalIdentifier.vi"("error in (no error)"=w1508, "local ID"=w1509, "diag ref in"=w1510) -> ("error out"=w1507:errorcluster, "success?"=w1506:bool, "data out"=w1505:u8[], "diag ref out"=w1504:T19)  [unwired: 5 in]
              }
              frame "User-Defined" {
              }
              frame "UDS" {
                n365 = call <vilib>:"UDS ReadDataByIdentifier.vi"("error in (no error)"=w1520, "ID"=w1515, "diag ref in"=w1519) -> ("error out"=w1518:errorcluster, "success?"=w1517:bool, "data out"=w1516:u8[], "diag ref out"=w1514:T19)  [unwired: 5 in]
              }
            }
            n366 = call "Signals.Scale.EU.vi"("Buffer?"=w1481, "Type"=w1485, "Lookup"=w1492, "error in (no error)"=w1489, "Unscaled Data"=w1490, "ID"=w1484, "Reads Ref"=w1488) -> ("error out"=w1487:errorcluster)  [unwired: 4 in]
            n367 = call "ServiceChannels.Status.Set.vi"("Buffer?"=w1481, "Type"=w1485, "Status Lookup"=w1482, "error in (no error)"=w1487, "ID"=w1484, "Service Channels Status Ref"=w1483) -> ("error out"=w1486:errorcluster)  [unwired: 5 in]
          }
          n368 = And Array Elements(Boolean array=w1476) -> (logical AND=w1470:bool)
          n369 = call "Status.Set.vi"("error in (no error)"=w1471, "success?"=w1470, "Data"=w1467, "Status Ref"=w1469) -> ("error out"=w1468:errorcluster)  [unwired: 7 in]
          n370 = call-poly <vilib>:"Data.Processes.Execute.vi"("error in (no error)"=w1468, "Ref"=w1466) -> ("error out"=w1452:errorcluster)  [unwired: 9 in]
          n371 = flat-sequence {
            tunnel: w1454 -> [w1480]
            tunnel: w1452 -> [w1479]
            tunnel: [w1477] -> w1451
            frame #0 {
              n372 = call-poly <vilib>:"Data.Processes.Execute.vi"("Ref"=w1480) -> ("error out"=w1478:errorcluster)  [unwired: 10 in]
              n373 = Merge Errors(w1479, w1478) -> (w1477:errorcluster)
            }
          }
          n374 = in-place-cluster #27("Status"=w1469, "Parameters.Properties.Service Channels Status Lookup"=w1453, "Service Channels Status"=w1454, "Reads"=w1466, "ADCS Connection"=w1473, "Parameters.Properties.Frames Lookup"=w1475, "Parameters.Properties.CAN.Diagnostic Protocol"=w1472) -> (w1447:T1)
          n375 = in-place-cluster #26("Polling.Queued"=w1455) -> (w1444:T31)
        }
      }
      frame "ReadDIDs" {
        n376 = in-place {
          in-place-border: w1525 -> [w1542]
          in-place-border: [w1526] -> w1524
          in-place-border: w1521 -> [w1536]
          n377 = in-place-cluster #28(w1523) -> ("Status"=w1533:T26, "Service Channels Status"=w1528:T26, "Parameters.Properties.Service Channels Status Lookup"=w1529:variant, "Reads"=w1530:T26, "ADCS Connection"=w1539:T19, "Parameters.Properties.Frames Lookup"=w1540:variant, "Parameters.Properties.CAN.Diagnostic Protocol"=w1537:T6)
          n378 = Unbundle By Name(w1536) -> ("DID IDs"=w1541:u32[])
          n379 = for {
            shift-right: [w1552] -> w1535
            shift-left: w1542 -> [w1563]
            shift-right: [w1558] -> w1538
            shift-left: w1539 -> [w1560]
            tunnel: w1540 -> [w1559]
            tunnel: w1541 -> [w1550] mode=indexing
            tunnel: [w1562] -> w1543 mode=indexing
            tunnel: w1537 -> [w1561]
            tunnel: [w1557] -> w1531
            tunnel: w1530 -> [w1555]
            tunnel: w1528 -> [w1549]
            tunnel: w1529 -> [w1548]
            stop <- w1552 stop-if-true
            w1551 = TRUE ("Buffer?")
            w1554 = Type."DID" ("Type")
            n380 = case shown="\"UDS\"" w1561 {
              tunnel: w1563 -> [w1567 w1575 w1580 w1587]
              tunnel: w1560 -> [w1569 w1577 w1579 w1586]
              tunnel: [w1565 w1574 w1580 w1585] -> w1556
              tunnel: [w1570 w1573 FALSE ("success?") w1584] -> w1562
              tunnel: [w1564 w1572 _ w1583] -> w1557
              tunnel: w1550 -> [w1566 w1576 _ w1582]
              tunnel: [w1568 w1571 w1579 w1581] -> w1558
              frame "GMLAN", Default {
                n381 = call "GMLAN ReadDataByIdentifier.vi"("error in (no error)"=w1567, "Data ID (DID)"=w1566, "diag ref in"=w1569) -> ("error out"=w1565:errorcluster, "success?"=w1570:bool, "data out"=w1564:u8[], "diag ref out"=w1568:T19)  [unwired: 5 in]
              }
              frame "KWP-2000" {
                n382 = call <vilib>:"ReadDataByLocalIdentifier.vi"("error in (no error)"=w1575, "local ID"=w1576, "diag ref in"=w1577) -> ("error out"=w1574:errorcluster, "success?"=w1573:bool, "data out"=w1572:u8[], "diag ref out"=w1571:T19)  [unwired: 5 in]
              }
              frame "User-Defined" {
              }
              frame "UDS" {
                n383 = call <vilib>:"UDS ReadDataByIdentifier.vi"("error in (no error)"=w1587, "ID"=w1582, "diag ref in"=w1586) -> ("error out"=w1585:errorcluster, "success?"=w1584:bool, "data out"=w1583:u8[], "diag ref out"=w1581:T19)  [unwired: 5 in]
              }
            }
            n384 = call "Signals.Scale.EU.vi"("Buffer?"=w1551, "Type"=w1554, "Lookup"=w1559, "error in (no error)"=w1556, "Unscaled Data"=w1557, "ID"=w1550, "Reads Ref"=w1555) -> ("error out"=w1553:errorcluster)  [unwired: 4 in]
            n385 = call "ServiceChannels.Status.Set.vi"("Buffer?"=w1551, "Type"=w1554, "Status Lookup"=w1548, "error in (no error)"=w1553, "ID"=w1550, "Service Channels Status Ref"=w1549) -> ("error out"=w1552:errorcluster)  [unwired: 5 in]
          }
          n386 = And Array Elements(Boolean array=w1543) -> (logical AND=w1534:bool)
          n387 = call "Status.Set.vi"("error in (no error)"=w1535, "success?"=w1534, "Data"=w1531, "Status Ref"=w1533) -> ("error out"=w1532:errorcluster)  [unwired: 7 in]
          n388 = call-poly <vilib>:"Data.Processes.Execute.vi"("error in (no error)"=w1532, "Ref"=w1530) -> ("error out"=w1527:errorcluster)  [unwired: 9 in]
          n389 = flat-sequence {
            tunnel: w1528 -> [w1547]
            tunnel: w1527 -> [w1546]
            tunnel: [w1544] -> w1526
            frame #0 {
              n390 = call-poly <vilib>:"Data.Processes.Execute.vi"("Ref"=w1547) -> ("error out"=w1545:errorcluster)  [unwired: 10 in]
              n391 = Merge Errors(w1546, w1545) -> (w1544:errorcluster)
            }
          }
          n392 = in-place-cluster #28("Status"=w1533, "Service Channels Status"=w1528, "Parameters.Properties.Service Channels Status Lookup"=w1529, "Reads"=w1530, "ADCS Connection"=w1538, "Parameters.Properties.Frames Lookup"=w1540, "Parameters.Properties.CAN.Diagnostic Protocol"=w1537) -> (w1522:T1)
        }
      }
      frame "ReadDID" {
        n393 = in-place {
          in-place-border: w1595 -> [w1622]
          in-place-border: w1594 -> [w1621]
          in-place-border: w1596 -> [_]
          in-place-border: [w1611] -> w1593
          in-place-border: w1589 -> [w1610]
          in-place-border: w1588 -> [w1609]
          w1600 = Type."DID" ("Type")
          n394 = in-place-cluster #29(w1592) -> ("Status"=w1616:T26, "Parameters.Properties.Service Channels Status Lookup"=w1597:variant, "Service Channels Status"=w1598:T26, "Reads"=w1615:T26, "ADCS Connection"=w1619:T19, "Parameters.Properties.Frames Lookup"=w1620:variant, "Parameters.Properties.CAN.Diagnostic Protocol"=w1617:T6)
          n395 = Unflatten From String(type=u16 0 ("ID"), binary string=w1621, error in (no error)=w1622) -> (value=w1599:u16, error out=w1623:errorcluster)  [unwired: 2 in, 1 out]
          n396 = case shown="\"User-Defined\"" w1617 {
            tunnel: w1623 -> [w1627 w1635 w1640 w1647]
            tunnel: w1619 -> [w1629 w1637 w1639 w1646]
            tunnel: [w1625 w1634 w1640 w1645] -> w1613
            tunnel: [w1630 w1633 FALSE ("success?") w1644] -> w1612
            tunnel: [w1624 w1632 _ w1643] -> w1607
            tunnel: w1599 -> [w1626 w1636 _ w1642]
            tunnel: [w1628 w1631 w1639 w1641] -> w1618
            frame "GMLAN", Default {
              n397 = call "GMLAN ReadDataByIdentifier.vi"("error in (no error)"=w1627, "Data ID (DID)"=w1626, "diag ref in"=w1629) -> ("error out"=w1625:errorcluster, "success?"=w1630:bool, "data out"=w1624:u8[], "diag ref out"=w1628:T19)  [unwired: 5 in]
            }
            frame "KWP-2000" {
              n398 = call <vilib>:"ReadDataByLocalIdentifier.vi"("error in (no error)"=w1635, "local ID"=w1636, "diag ref in"=w1637) -> ("error out"=w1634:errorcluster, "success?"=w1633:bool, "data out"=w1632:u8[], "diag ref out"=w1631:T19)  [unwired: 5 in]
            }
            frame "User-Defined" {
            }
            frame "UDS" {
              n399 = call <vilib>:"UDS ReadDataByIdentifier.vi"("error in (no error)"=w1647, "ID"=w1642, "diag ref in"=w1646) -> ("error out"=w1645:errorcluster, "success?"=w1644:bool, "data out"=w1643:u8[], "diag ref out"=w1641:T19)  [unwired: 5 in]
            }
          }
          n400 = call "Signals.Scale.EU.vi"("Type"=w1600, "Lookup"=w1620, "error in (no error)"=w1613, "Unscaled Data"=w1607, "ID"=w1599, "Reads Ref"=w1615) -> ("error out"=w1602:errorcluster)  [unwired: 5 in]
          n401 = call "ServiceChannels.Status.Set.vi"("Type"=w1600, "Status Lookup"=w1597, "error in (no error)"=w1602, "ID"=w1599, "Service Channels Status Ref"=w1598) -> ("error out"=w1601:errorcluster)  [unwired: 6 in]
          n402 = Bundle By Name(cluster=T36 {"ID"=0, "Raw Frame"=[], "error out"={"status"=FALSE, "code"=0, "source"=""}}, "ID"=w1599, "Raw Frame"=w1607) -> (w1605:T36)
          n403 = Flatten To String(anything=w1605, error in (no error)=w1601) -> (data string=w1604:string, error out=w1606:errorcluster)  [unwired: 2 in, 1 out]
          n404 = call "Status.Set.vi"("error in (no error)"=w1606, "success?"=w1612, "Data"=w1607, "Status Ref"=w1616) -> ("error out"=w1603:errorcluster)  [unwired: 7 in]
          n405 = in-place-cluster #29("Status"=w1616, "Parameters.Properties.Service Channels Status Lookup"=w1597, "Service Channels Status"=w1598, "Reads"=w1615, "ADCS Connection"=w1618, "Parameters.Properties.Frames Lookup"=w1620, "Parameters.Properties.CAN.Diagnostic Protocol"=w1617) -> (w1591:T1)
          n406 = call <vilib>:"Respond to Command.vi"("error in (no error)"=w1603, "message value"=w1604, "ResponseInfo"=w1610, "VeriStand Comm in"=w1609) -> ("error out"=w1611:errorcluster)  [unwired: 5 in, 2 out]
        }
      }
      frame "GenerateCDID" {
        n407 = in-place {
          in-place-border: w1652 -> [w1673]
          in-place-border: w1651 -> [w1672]
          in-place-border: [w1664] -> w1650
          w1656 = Type."CDID" ("Type")
          n408 = in-place-cluster #30(w1649) -> ("Status"=w1662:T26, "Parameters.Properties.Service Channels Status Lookup"=w1654:variant, "Service Channels Status"=w1655:T26, "ADCS Connection"=w1671:T19, "Parameters.Properties.CAN.Diagnostic Protocol"=w1669:T6, "Parameters.Properties.Frames Lookup"=w1665:variant, "Writes"=w1661:T27)
          n409 = Unflatten From String(type=u16 0, binary string=w1672, error in (no error)=w1673) -> (value=w1657:u16, error out=w1660:errorcluster)  [unwired: 2 in, 1 out]
          n410 = call "Signals.Scale.Raw.vi"("Type"=w1656, "Lookup"=w1665, "error in"=w1660, "ID"=w1657, "Writes Ref"=w1661) -> ("error out"=w1667:errorcluster, "Data"=w1666:u8[])  [unwired: 5 in]
          n411 = case shown="\"KWP-2000\"" w1669 {
            tunnel: w1657 -> [w1679 w1681 _ w1691]
            tunnel: w1666 -> [w1677 w1682 _ w1692]
            tunnel: [w1676 w1684 w1689 w1697] -> w1659
            tunnel: [w1675 w1683 FALSE ("success?") w1696] -> w1663
            tunnel: w1667 -> [w1680 w1685 w1689 w1695]
            tunnel: w1671 -> [w1678 w1687 w1690 w1694]
            tunnel: [w1674 w1686 w1690 w1693] -> w1670
            frame "KWP-2000" {
              n412 = call <vilib>:"WriteDataByLocalIdentifier.vi"("data in"=w1677, "error in (no error)"=w1680, "local ID"=w1679, "diag ref in"=w1678) -> ("error out"=w1676:errorcluster, "success?"=w1675:bool, "diag ref out"=w1674:T19)  [unwired: 5 in]
            }
            frame "GMLAN" {
              n413 = call "GMLAN WriteDataByIdentifier.vi"("error in (no error)"=w1685, "data"=w1682, "Data ID (DID)"=w1681, "diag ref in"=w1687) -> ("error out"=w1684:errorcluster, "success?"=w1683:bool, "diag ref out"=w1686:T19)  [unwired: 5 in]
            }
            frame "User-Defined" {
            }
            frame "UDS" {
              n414 = call <vilib>:"UDS WriteDataByIdentifier.vi"("data in"=w1692, "error in (no error)"=w1695, "ID"=w1691, "diag ref in"=w1694) -> ("error out"=w1697:errorcluster, "success?"=w1696:bool, "diag ref out"=w1693:T19)  [unwired: 5 in]
            }
          }
          n415 = call "ServiceChannels.Status.Set.vi"("Type"=w1656, "Status Lookup"=w1654, "error in (no error)"=w1659, "ID"=w1657, "Service Channels Status Ref"=w1655) -> ("error out"=w1658:errorcluster)  [unwired: 6 in]
          n416 = call "Status.Set.vi"("error in (no error)"=w1658, "success?"=w1663, "Status Ref"=w1662) -> ("error out"=w1664:errorcluster)  [unwired: 8 in]
          n417 = in-place-cluster #30("Status"=w1662, "Parameters.Properties.Service Channels Status Lookup"=w1654, "Service Channels Status"=w1655, "ADCS Connection"=w1670, "Parameters.Properties.CAN.Diagnostic Protocol"=w1669, "Parameters.Properties.Frames Lookup"=w1665, "Writes"=w1661) -> (w1648:T1)
        }
      }
      frame "ChannelPassThru" {
        n418 = in-place {
          in-place-border: w1704 -> [_]
          in-place-border: [w1714] -> w1703
          in-place-border: w1702 -> [_]
          in-place-border: w1701 -> [w1731]
          in-place-border: w1700 -> [w1730]
          n419 = in-place-cluster #31(w1699) -> ("Status"=w1708:T26, "ADCS Connection"=w1728:T19)
          n420 = Unflatten From String(type=T45 {"Service"=0, "Service Length"=0, "Data Length"=0, "Response Required"=FALSE}, binary string=w1731, error in (no error)=w1730) -> (value=w1729:T45, error out=w1710:errorcluster)  [unwired: 2 in, 1 out]
          n421 = Unbundle By Name(w1729) -> ("Response Required"=w1715:bool, "Service"=w1724:u64, "Service Length"=w1721:u8, "Data Length"=w1720:u32)
          n422 = Type Cast(type=u8[] [], x=w1724) -> (*(type *) &x=w1722:u8[])
          n423 = Subtract(x=u8 8 ("y"), y=w1721) -> (x-y=w1706:u8)
          n424 = Array Subset(array=w1722, index=w1706) -> (w1718:u8[])  [unwired: 1 in]
          n425 = Initialize Array(u8 0, w1720) -> (w1717:u8[])
          n426 = Build Array (concatenate)(w1718, w1717) -> (w1716:u8[])
          n427 = call <vilib>:"Diagnostic Service.vi"("error source"="Diagnostic Service.vi", "error in (no error)"=w1710, "data in"=w1716, "require response?"=w1715, "diag ref in"=w1728) -> ("error out"=w1709:errorcluster, "data out"=w1713:u8[], "error code"=w1712:u8, "diag ref out"=w1727:T19)  [unwired: 1 in, 2 out]
          n428 = Equal To 0?(x=w1712) -> (x = 0?=w1711:bool)
          n429 = call "Status.Set.vi"("error in (no error)"=w1709, "success?"=w1711, "Data"=w1713, "Status Ref"=w1708) -> ("error out"=w1714:errorcluster)  [unwired: 7 in]
          n430 = in-place-cluster #31("Status"=w1708, "ADCS Connection"=w1727) -> (w1698:T1)
        }
      }
      frame "UserDefinedMessage" {
        n431 = in-place {
          in-place-border: w1736 -> [w1764]
          in-place-border: [w1745] -> w1732
          in-place-border: w1735 -> [w1763]
          w1738 = Type."User Defined" ("Type")
          n432 = in-place-cluster #32(w1734) -> ("Status"=w1762:T26, "Parameters.Properties.Service Channels Status Lookup"=w1740:variant, "Service Channels Status"=w1741:T26, "Parameters.Properties.Frames Lookup"=w1755:variant, "Reads"=w1744:T26, "ADCS Connection"=w1760:T19, "Writes"=w1746:T27)
          n433 = Unflatten From String(type=u32 0 ("ID"), binary string=w1763, error in (no error)=w1764) -> (value=w1739:u32, error out=w1747:errorcluster)  [unwired: 2 in, 1 out]
          n434 = call "Signals.Scale.Raw.vi"("Type"=w1738, "Lookup"=w1755, "error in"=w1747, "ID"=w1739, "Writes Ref"=w1746) -> ("error out"=w1754:errorcluster, "Data"=w1759:u8[])  [unwired: 5 in]
          n435 = call "Frames.Lookup.Size.Get.vi"("Type"=w1738, "error in (no error)"=w1754, "ID"=w1739, "Frames Lookup"=w1755) -> ("error out"=w1753:errorcluster, "ByteLength"=w1749:u16)  [unwired: 5 in, 1 out]
          n436 = Not Equal To 0?(x=w1749) -> (x != 0?=w1752:bool)
          n437 = disable-structure shown="Default" {
            disable-tunnel: w1760 -> [w1773 w1777]
            disable-tunnel: w1759 -> [w1772 w1775]
            disable-tunnel: [w1771 w1781] -> w1750
            disable-tunnel: [w1770 w1778] -> w1758
            disable-tunnel: [w1769 w1780] -> w1748
            disable-tunnel: [w1768 w1779] -> w1757
            disable-tunnel: w1753 -> [w1767 w1782]
            disable-tunnel: w1752 -> [w1766 w1776]
            disable-tunnel: "Diagnostic Service.vi" ("error source") -> [w1765 w1774]
            frame condition #0 (active) {
              n438 = call <vilib>:"Diagnostic Service.vi"("error source"=w1765, "error in (no error)"=w1767, "data in"=w1772, "require response?"=w1766, "diag ref in"=w1773) -> ("error out"=w1771:errorcluster, "data out"=w1769:u8[], "error code"=w1768:u8, "diag ref out"=w1770:T19)  [unwired: 1 in, 2 out]
            }
            frame condition #1 {
              n439 = call "CustomerSpecific_SendReceive.vi"("error source"=w1774, "error in (no error)"=w1782, "data in"=w1775, "require response?"=w1776, "diag ref in"=w1777) -> ("error out"=w1781:errorcluster, "data out"=w1780:u8[], "error code"=w1779:u8, "diag ref out"=w1778:T19)  [unwired: 3 in]
            }
          }
          n440 = Equal To 0?(x=w1757) -> (x = 0?=w1756:bool)
          n441 = call "Signals.Scale.EU.vi"("Type"=w1738, "Lookup"=w1755, "error in (no error)"=w1750, "Unscaled Data"=w1748, "ID"=w1739, "Reads Ref"=w1744) -> ("error out"=w1743:errorcluster)  [unwired: 5 in]
          n442 = call "ServiceChannels.Status.Set.vi"("Type"=w1738, "Status Lookup"=w1740, "error in (no error)"=w1743, "ID"=w1739, "Service Channels Status Ref"=w1741) -> ("error out"=w1742:errorcluster)  [unwired: 6 in]
          n443 = in-place-cluster #32("Status"=w1762, "Parameters.Properties.Service Channels Status Lookup"=w1740, "Service Channels Status"=w1741, "Parameters.Properties.Frames Lookup"=w1755, "Reads"=w1744, "ADCS Connection"=w1758, "Writes"=w1746) -> (w1733:T1)
          n444 = call "Status.Set.vi"("error in (no error)"=w1742, "success?"=w1756, "Data"=w1748, "Status Ref"=w1762) -> ("error out"=w1745:errorcluster)  [unwired: 7 in]
        }
      }
      frame "<--------------- TCP ONLY --------------->" {
      }
      frame "PassThru" {
        n445 = in-place {
          in-place-border: w1792 -> [w1795]
          in-place-border: [w1813] -> w1791
          in-place-border: w1790 -> [w1808]
          in-place-border: w1789 -> [w1807]
          in-place-border: w1786 -> [w1794]
          n446 = in-place-cluster #33(w1788) -> ("ADCS Connection"=w1804:T19)
          n447 = Unflatten From String(type=cluster{"cmd":u8[], "require response?":bool} {"cmd"=[], "require response?"=TRUE}, binary string=w1808, error in (no error)=w1807) -> (value=w1805:cluster{"cmd":u8[], "require response?":bool}, error out=w1801:errorcluster)  [unwired: 2 in, 1 out]
          n448 = Unbundle By Name(w1805) -> ("require response?"=w1803:bool, "cmd"=w1802:u8[])
          n449 = disable-structure shown="Default" {
            disable-tunnel: w1804 -> [w1822 w1826]
            disable-tunnel: w1802 -> [w1821 w1824]
            disable-tunnel: [w1820 w1830] -> w1800
            disable-tunnel: [w1819 w1827] -> w1797
            disable-tunnel: [w1818 w1829] -> w1799
            disable-tunnel: [w1817 w1828] -> w1798
            disable-tunnel: w1801 -> [w1816 w1831]
            disable-tunnel: w1803 -> [w1815 w1825]
            disable-tunnel: "Diagnostic Service.vi" ("error source") -> [w1814 w1823]
            frame condition #0 (active) {
              n450 = call <vilib>:"Diagnostic Service.vi"("error source"=w1814, "error in (no error)"=w1816, "data in"=w1821, "require response?"=w1815, "diag ref in"=w1822) -> ("error out"=w1820:errorcluster, "data out"=w1818:u8[], "error code"=w1817:u8, "diag ref out"=w1819:T19)  [unwired: 1 in, 2 out]
            }
            frame condition #1 {
              n451 = call "CustomerSpecific_SendReceive.vi"("error source"=w1823, "error in (no error)"=w1831, "data in"=w1824, "require response?"=w1825, "diag ref in"=w1826) -> ("error out"=w1830:errorcluster, "data out"=w1829:u8[], "error code"=w1828:u8, "diag ref out"=w1827:T19)  [unwired: 3 in]
            }
          }
          n452 = Bundle By Name(cluster=T46 {"resp"=[], "error code"=0, "error out"={"status"=FALSE, "code"=0, "source"=""}}, "error code"=w1798, "resp"=w1799, "error out"=w1800) -> (w1810:T46)
          n453 = Flatten To String(anything=w1810, error in (no error)=w1801) -> (data string=w1809:string, error out=w1811:errorcluster)  [unwired: 2 in, 1 out]
          n454 = in-place-cluster #33("ADCS Connection"=w1797) -> (w1787:T1)
          n455 = call <vilib>:"Respond to Command.vi"("error in (no error)"=w1811, "message value"=w1809, "ResponseInfo"=w1795, "VeriStand Comm in"=w1794) -> ("error out"=w1813:errorcluster)  [unwired: 5 in, 2 out]
        }
      }
      frame "<--------------- UDS/KWP ONLY --------------->" {
      }
      frame "ControlDTC" {
        n456 = in-place {
          in-place-border: w1837 -> [w1859]
          in-place-border: [w1849] -> w1836
          in-place-border: w1835 -> [w1858]
          n457 = in-place-cluster #34(w1839) -> ("Status"=w1848:T26, "Parameters.Properties.DTC.Descriptor"=w1842:T17, "Parameters.Properties.Frames Lookup"=w1852:variant, "ADCS Connection"=w1861:T19, "Parameters.Properties.CAN.Diagnostic Protocol"=w1862:T6, "Writes"=w1847:T27)
          n458 = Unflatten From String(type=T47 {"Group/Type"=16777215, "Byte Lengths (KWP only)"={"Override"=FALSE, "DTC"=0, "Status"=0, "Failure"=0}} ("Clear DTC Settings"), binary string=w1858, error in (no error)=w1859) -> (value=w1857:T47, error out=w1846:errorcluster)  [unwired: 2 in, 1 out]
          n459 = Unbundle By Name(w1857) -> ("Byte Lengths (KWP only)"=w1843:T43, "Group/Type"=w1844:u32)
          n460 = call "DTC.Descriptor.Override.vi"("Byte Lengths"=w1843, "Descriptor in"=w1842) -> ("Descriptor out"=w1841:T17)  [unwired: 9 in]
          n461 = call "Signals.Scale.Raw.vi"("Type"=Type."DTC Control", "Lookup"=w1852, "error in"=w1846, "ID"=u32 0, "Writes Ref"=w1847) -> ("error out"=w1855:errorcluster, "Data"=w1853:u8[])  [unwired: 5 in]
          n462 = case shown="\"UDS\"" w1862 {
            tunnel: w1855 -> [w1865 w1872 w1880]
            tunnel: [w1865 w1871 w1879] -> w1851
            tunnel: w1841 -> [_ _ w1878]
            tunnel: w1861 -> [w1864 w1869 w1877]
            tunnel: [w1864 w1870 w1876] -> w1860
            tunnel: [FALSE ("success?") w1868 w1875] -> w1850
            tunnel: w1844 -> [_ w1867 w1874]
            tunnel: w1853 -> [_ w1866 w1873]
            frame "GMLAN", "User-Defined" {
            }
            frame "UDS" {
              n463 = call <vilib>:"UDS ControlDTCSetting.vi"("error in (no error)"=w1872, "type"=w1867, "data in"=w1866, "diag ref in"=w1869) -> ("error out"=w1871:errorcluster, "success?"=w1868:bool, "diag ref out"=w1870:T19)  [unwired: 5 in]
            }
            frame "KWP-2000" {
              n464 = call <vilib>:"ControlDTCSetting.vi"("DTC descriptor"=w1878, "error in (no error)"=w1880, "group of DTC"=w1874, "data in"=w1873, "diag ref in"=w1877) -> ("error out"=w1879:errorcluster, "success?"=w1875:bool, "diag ref out"=w1876:T19)  [unwired: 4 in]
            }
          }
          n465 = call "Status.Set.vi"("error in (no error)"=w1851, "success?"=w1850, "Status Ref"=w1848) -> ("error out"=w1849:errorcluster)  [unwired: 8 in]
          n466 = in-place-cluster #34("Status"=w1848, "Parameters.Properties.DTC.Descriptor"=w1842, "Parameters.Properties.Frames Lookup"=w1852, "ADCS Connection"=w1860, "Parameters.Properties.CAN.Diagnostic Protocol"=w1862, "Writes"=w1847) -> (w1838:T1)
        }
      }
      frame "ECUReset" {
        n467 = in-place {
          in-place-border: w1885 -> [w1895]
          in-place-border: [w1888] -> w1884
          in-place-border: w1883 -> [w1894]
          n468 = in-place-cluster #35(w1882) -> ("Status"=w1887:T26, "Parameters.Properties.CAN.Diagnostic Protocol"=w1891:T6, "ADCS Connection"=w1893:T19)
          n469 = Unflatten From String(type=u8 0 ("ID"), binary string=w1894, error in (no error)=w1895) -> (value=w1898:u8, error out=w1897:errorcluster)  [unwired: 2 in, 1 out]
          n470 = case shown="\"GMLAN\", \"User-Defined\"" w1891 {
            tunnel: [FALSE ("success?") w1905 w1913] -> w1889
            tunnel: [w1900 w1906 w1912] -> w1890
            tunnel: w1898 -> [_ w1902 w1911]
            tunnel: w1897 -> [w1900 w1907 w1910]
            tunnel: w1893 -> [w1901 w1903 w1909]
            tunnel: [w1901 w1904 w1908] -> w1892
            frame "GMLAN", "User-Defined" {
            }
            frame "KWP-2000" {
              n471 = call <vilib>:"ECUReset.vi"("error in (no error)"=w1907, "mode"=w1902, "diag ref in"=w1903) -> ("error out"=w1906:errorcluster, "success?"=w1905:bool, "diag ref out"=w1904:T19)  [unwired: 6 in]
            }
            frame "UDS" {
              n472 = call <vilib>:"UDS ECUReset.vi"("error in (no error)"=w1910, "mode"=w1911, "diag ref in"=w1909) -> ("error out"=w1912:errorcluster, "success?"=w1913:bool, "diag ref out"=w1908:T19)  [unwired: 5 in, 1 out]
            }
          }
          n473 = call "Status.Set.vi"("error in (no error)"=w1890, "success?"=w1889, "Status Ref"=w1887) -> ("error out"=w1888:errorcluster)  [unwired: 8 in]
          n474 = in-place-cluster #35("Status"=w1887, "Parameters.Properties.CAN.Diagnostic Protocol"=w1891, "ADCS Connection"=w1892) -> (w1881:T1)
        }
      }
      frame "ReadMemory" {
        n475 = in-place {
          in-place-border: w1918 -> [w1937]
          in-place-border: [w1929] -> w1917
          in-place-border: w1916 -> [w1936]
          w1923 = Type."Read Memory" ("Type")
          n476 = in-place-cluster #36(w1915) -> ("Status"=w1930:T26, "Parameters.Properties.CAN.Diagnostic Protocol"=w1939:T6, "Parameters.Properties.Service Channels Status Lookup"=w1920:variant, "Service Channels Status"=w1921:T26, "Parameters.Properties.Frames Lookup"=w1932:variant, "Reads"=w1926:T26, "ADCS Connection"=w1940:T19)
          n477 = Unflatten From String(type=T48 {"Address"=0, "Service Type"=0, "Address Length"=0, "Size Length"=0}, binary string=w1936, error in (no error)=w1937) -> (value=w1934:T48, error out=w1933:errorcluster)  [unwired: 2 in, 1 out]
          n478 = case shown="\"UDS\"" w1939 {
            tunnel: [w1949 w1965 w1987] -> w1935
            tunnel: [w1951 w1966 w1986] -> w1938
            tunnel: w1933 -> [w1946 w1955 w1987]
            tunnel: w1940 -> [w1952 w1967 w1986]
            tunnel: [w1948 w1964 _] -> w1931
            tunnel: w1934 -> [w1947 w1962 _]
            tunnel: [w1950 w1963 _] -> w1928
            tunnel: w1932 -> [w1944 w1958 _]
            tunnel: [w1943 w1953 _] -> w1922
            frame "KWP-2000" {
              n479 = Unbundle By Name(w1947) -> ("Address"=w1943:u64)
              n480 = call "Frames.Lookup.Size.Get.vi"("Type"=Type."Read Memory", "error in (no error)"=w1946, "ID"=w1943, "Frames Lookup"=w1944) -> ("error out"=w1945:errorcluster, "ByteLength"=w1942:u16)  [unwired: 5 in, 1 out]
              n481 = call <vilib>:"ReadMemoryByAddress.vi"("error in (no error)"=w1945, "size"=w1942, "address"=w1943, "diag ref in"=w1952) -> ("error out"=w1949:errorcluster, "success?"=w1948:bool, "data out"=w1950:u8[], "diag ref out"=w1951:T19)  [unwired: 4 in]
            }
            frame "UDS" {
              n482 = Unbundle By Name(w1962) -> ("Service Type"=w1961:u32, "Address"=w1953:u64, "Address Length"=w1960:u8, "Size Length"=w1959:u8)
              n483 = call "Frames.Lookup.Size.Get.vi"("Type"=Type."Read Memory", "error in (no error)"=w1955, "ID"=w1953, "Frames Lookup"=w1958) -> ("error out"=w1954:errorcluster, "ByteLength"=w1956:u16)  [unwired: 5 in, 1 out]
              n484 = case shown="1, Default" w1961 {
                tunnel: w1967 -> [w1977 w1985]
                tunnel: [w1973 w1984] -> w1966
                tunnel: w1954 -> [w1976 w1983]
                tunnel: [w1975 w1982] -> w1965
                tunnel: [w1972 w1981] -> w1964
                tunnel: [w1974 w1980] -> w1963
                tunnel: w1953 -> [w1969 w1979]
                tunnel: w1960 -> [w1971 _]
                tunnel: w1959 -> [w1970 _]
                tunnel: w1956 -> [w1968 w1978]
                frame 2 {
                  n485 = call <vilib>:"UDS06 ReadMemoryByAddress.vi"("memory size length"=w1970, "memory address length"=w1971, "error in (no error)"=w1976, "memory size"=w1968, "memory address"=w1969, "diag ref in"=w1977) -> ("error out"=w1975:errorcluster, "success?"=w1972:bool, "data out"=w1974:u8[], "diag ref out"=w1973:T19)  [unwired: 2 in]
                }
                frame 1, Default {
                  n486 = call <vilib>:"UDS ReadMemoryByAddress.vi"("error in (no error)"=w1983, "size"=w1978, "address"=w1979, "diag ref in"=w1985) -> ("error out"=w1982:errorcluster, "success?"=w1981:bool, "data out"=w1980:u8[], "diag ref out"=w1984:T19)  [unwired: 4 in]
                }
              }
            }
            frame "GMLAN", "User-Defined" {
            }
          }
          n487 = call "Signals.Scale.EU.vi"("Type"=w1923, "Lookup"=w1932, "error in (no error)"=w1935, "Unscaled Data"=w1928, "ID"=w1922, "Reads Ref"=w1926) -> ("error out"=w1925:errorcluster)  [unwired: 5 in]
          n488 = call "ServiceChannels.Status.Set.vi"("Type"=w1923, "Status Lookup"=w1920, "error in (no error)"=w1925, "ID"=w1922, "Service Channels Status Ref"=w1921) -> ("error out"=w1924:errorcluster)  [unwired: 6 in]
          n489 = call "Status.Set.vi"("error in (no error)"=w1924, "success?"=w1931, "Data"=w1928, "Status Ref"=w1930) -> ("error out"=w1929:errorcluster)  [unwired: 7 in]
          n490 = in-place-cluster #36("Status"=w1930, "Parameters.Properties.CAN.Diagnostic Protocol"=w1939, "Parameters.Properties.Service Channels Status Lookup"=w1920, "Service Channels Status"=w1921, "Parameters.Properties.Frames Lookup"=w1932, "Reads"=w1926, "ADCS Connection"=w1938) -> (w1914:T1)
        }
      }
      frame "WriteMemory" {
        n491 = in-place {
          in-place-border: w1992 -> [w2014]
          in-place-border: [w2008] -> w1991
          in-place-border: w1990 -> [w2013]
          w1994 = Type."Write Memory" ("Type")
          n492 = in-place-cluster #37(w1989) -> ("Status"=w2009:T26, "Parameters.Properties.CAN.Diagnostic Protocol"=w2016:T6, "Parameters.Properties.Service Channels Status Lookup"=w1996:variant, "Service Channels Status"=w1997:T26, "ADCS Connection"=w2017:T19, "Parameters.Properties.Frames Lookup"=w2004:variant, "Writes"=w2000:T27)
          n493 = Unflatten From String(type=T48 {"Address"=0, "Service Type"=0, "Address Length"=0, "Size Length"=0}, binary string=w2013, error in (no error)=w2014) -> (value=w2010:T48, error out=w2001:errorcluster)  [unwired: 2 in, 1 out]
          n494 = Unbundle By Name(w2010) -> ("Address"=w1995:u64, "Service Type"=w2005:u32, "Address Length"=w2003:u8, "Size Length"=w2002:u8)
          n495 = call "Signals.Scale.Raw.vi"("Type"=w1994, "Lookup"=w2004, "error in"=w2001, "ID"=w1995, "Writes Ref"=w2000) -> ("error out"=w2012:errorcluster, "Data"=w2011:u8[])  [unwired: 5 in]
          n496 = case shown="\"UDS\"" w2016 {
            tunnel: [w2023 w2035 w2056] -> w1999
            tunnel: [w2021 w2033 w2055] -> w2015
            tunnel: w2012 -> [w2024 w2036 w2056]
            tunnel: w2017 -> [w2025 w2032 w2055]
            tunnel: [w2022 w2034 _] -> w2007
            tunnel: w1995 -> [w2020 w2028 _]
            tunnel: w2011 -> [w2018 w2027 _]
            tunnel: w2005 -> [_ w2031 _]
            tunnel: w2004 -> [_ _ _]
            tunnel: w2003 -> [_ w2030 _]
            tunnel: w2002 -> [_ w2029 _]
            frame "KWP-2000" {
              n497 = Array Size(array=w2018) -> (size(s)=w2019:i32)
              n498 = call <vilib>:"WriteMemoryByAddress.vi"("data in"=w2018, "error in (no error)"=w2024, "size"=w2019, "address"=w2020, "diag ref in"=w2025) -> ("error out"=w2023:errorcluster, "success?"=w2022:bool, "diag ref out"=w2021:T19)  [unwired: 4 in]
            }
            frame "UDS" {
              n499 = Array Size(array=w2027) -> (size(s)=w2026:i32)
              n500 = case shown="2" w2031 {
                tunnel: w2036 -> [w2045 w2054]
                tunnel: [w2042 w2053] -> w2035
                tunnel: [w2041 w2052] -> w2034
                tunnel: [w2043 w2051] -> w2033
                tunnel: w2028 -> [w2040 w2050]
                tunnel: w2032 -> [w2046 w2049]
                tunnel: w2027 -> [w2044 w2048]
                tunnel: w2030 -> [w2039 _]
                tunnel: w2029 -> [w2038 _]
                tunnel: w2026 -> [w2037 w2047]
                frame 2 {
                  n501 = call <vilib>:"UDS06 WriteMemoryByAddress.vi"("memory size length"=w2038, "memory address length"=w2039, "data in"=w2044, "error in (no error)"=w2045, "memory size"=w2037, "memory address"=w2040, "diag ref in"=w2046) -> ("error out"=w2042:errorcluster, "success?"=w2041:bool, "diag ref out"=w2043:T19)  [unwired: 2 in]
                }
                frame 1, Default {
                  n502 = call <vilib>:"UDS WriteMemoryByAddress.vi"("data in"=w2048, "error in (no error)"=w2054, "size"=w2047, "address"=w2050, "diag ref in"=w2049) -> ("error out"=w2053:errorcluster, "success?"=w2052:bool, "diag ref out"=w2051:T19)  [unwired: 4 in]
                }
              }
            }
            frame "GMLAN", "User-Defined" {
            }
          }
          n503 = call "ServiceChannels.Status.Set.vi"("Type"=w1994, "Status Lookup"=w1996, "error in (no error)"=w1999, "ID"=w1995, "Service Channels Status Ref"=w1997) -> ("error out"=w1998:errorcluster)  [unwired: 6 in]
          n504 = call "Status.Set.vi"("error in (no error)"=w1998, "success?"=w2007, "Status Ref"=w2009) -> ("error out"=w2008:errorcluster)  [unwired: 8 in]
          n505 = in-place-cluster #37("Status"=w2009, "Parameters.Properties.CAN.Diagnostic Protocol"=w2016, "Parameters.Properties.Service Channels Status Lookup"=w1996, "Service Channels Status"=w1997, "ADCS Connection"=w2015, "Parameters.Properties.Frames Lookup"=w2004, "Writes"=w2000) -> (w1988:T1)
        }
      }
      frame "InputOutputControl" {
        n506 = in-place {
          in-place-border: w2061 -> [w2084]
          in-place-border: [w2073] -> w2059
          in-place-border: w2060 -> [w2083]
          w2063 = Type."IO Control" ("Type")
          n507 = in-place-cluster #38(w2058) -> ("Status"=w2074:T26, "Parameters.Properties.CAN.Diagnostic Protocol"=w2086:T6, "Parameters.Properties.Service Channels Status Lookup"=w2066:variant, "Service Channels Status"=w2065:T26, "Parameters.Properties.Frames Lookup"=w2076:variant, "Reads"=w2069:T26, "ADCS Connection"=w2087:T19, "Writes"=w2070:T27)
          n508 = Unflatten From String(type=T49 {"ID"=0, "Mode"=0}, binary string=w2083, error in (no error)=w2084) -> (value=w2078:T49, error out=w2071:errorcluster)  [unwired: 2 in, 1 out]
          n509 = Unbundle By Name(w2078) -> ("ID"=w2064:u16, "Mode"=w2077:u8)
          n510 = call "Signals.Scale.Raw.vi"("Type"=w2063, "Lookup"=w2076, "error in"=w2071, "ID"=w2064, "Writes Ref"=w2070) -> ("error out"=w2082:errorcluster, "Data"=w2081:u8[])  [unwired: 5 in]
          n511 = case shown="\"KWP-2000\"" w2086 {
            tunnel: [w2096 w2121 w2141] -> w2080
            tunnel: [w2095 w2117 w2140] -> w2085
            tunnel: w2082 -> [w2093 w2122 w2141]
            tunnel: w2087 -> [w2094 w2119 w2140]
            tunnel: [w2092 w2115 _] -> w2075
            tunnel: w2064 -> [w2091 w2120 _]
            tunnel: w2081 -> [w2090 w2118 _]
            tunnel: [w2089 w2116 _] -> w2072
            tunnel: w2077 -> [w2088 w2114 _]
            frame "KWP-2000" {
              n512 = case shown="Default" w2088 {
                selector: w2088 -> [w2097 w2106]
                tunnel: [w2105 w2113] -> w2096
                tunnel: [w2104 w2112] -> w2095
                tunnel: w2094 -> [w2103 w2111]
                tunnel: w2093 -> [w2102 w2110]
                tunnel: [w2101 w2109] -> w2092
                tunnel: w2091 -> [w2100 w2108]
                tunnel: w2090 -> [w2099 _]
                tunnel: [w2098 w2107] -> w2089
                frame Default {
                  n513 = call <vilib>:"InputOutputControlByLocalIdentifier.vi"("data in"=w2099, "error in (no error)"=w2102, "mode"=w2097, "local ID"=w2100, "diag ref in"=w2103) -> ("error out"=w2105:errorcluster, "success?"=w2101:bool, "data out"=w2098:u8[], "diag ref out"=w2104:T19)  [unwired: 3 in]
                }
                frame 0 {
                  n514 = call <vilib>:"InputOutputControlByLocalIdentifier.vi"("error in (no error)"=w2110, "mode"=w2106, "local ID"=w2108, "diag ref in"=w2111) -> ("error out"=w2113:errorcluster, "success?"=w2109:bool, "data out"=w2107:u8[], "diag ref out"=w2112:T19)  [unwired: 4 in]
                }
              }
            }
            frame "UDS" {
              n515 = case shown="Default" w2114 {
                selector: w2114 -> [w2123 w2131]
                tunnel: w2122 -> [w2128 w2139]
                tunnel: [w2127 w2138] -> w2121
                tunnel: w2120 -> [w2129 w2137]
                tunnel: w2119 -> [w2130 w2136]
                tunnel: w2118 -> [_ w2135]
                tunnel: [w2124 w2134] -> w2117
                tunnel: [w2125 w2133] -> w2116
                tunnel: [w2126 w2132] -> w2115
                frame 0 {
                  n516 = call <vilib>:"UDS InputOutputControlByIdentifier.vi"("error in (no error)"=w2128, "mode"=w2123, "ID"=w2129, "diag ref in"=w2130) -> ("error out"=w2127:errorcluster, "success?"=w2126:bool, "data out"=w2125:u8[], "diag ref out"=w2124:T19)  [unwired: 4 in]
                }
                frame Default {
                  n517 = call <vilib>:"UDS InputOutputControlByIdentifier.vi"("data in"=w2135, "error in (no error)"=w2139, "mode"=w2131, "ID"=w2137, "diag ref in"=w2136) -> ("error out"=w2138:errorcluster, "success?"=w2132:bool, "data out"=w2133:u8[], "diag ref out"=w2134:T19)  [unwired: 3 in]
                }
              }
            }
            frame "GMLAN", "User-Defined" {
            }
          }
          n518 = call "Signals.Scale.EU.vi"("Type"=w2063, "Lookup"=w2076, "error in (no error)"=w2080, "Unscaled Data"=w2072, "ID"=w2064, "Reads Ref"=w2069) -> ("error out"=w2068:errorcluster)  [unwired: 5 in]
          n519 = call "ServiceChannels.Status.Set.vi"("Type"=w2063, "Status Lookup"=w2066, "error in (no error)"=w2068, "ID"=w2064, "Service Channels Status Ref"=w2065) -> ("error out"=w2067:errorcluster)  [unwired: 6 in]
          n520 = call "Status.Set.vi"("error in (no error)"=w2067, "success?"=w2075, "Data"=w2072, "Status Ref"=w2074) -> ("error out"=w2073:errorcluster)  [unwired: 7 in]
          n521 = in-place-cluster #38("Status"=w2074, "Parameters.Properties.CAN.Diagnostic Protocol"=w2086, "Parameters.Properties.Service Channels Status Lookup"=w2066, "Service Channels Status"=w2065, "Parameters.Properties.Frames Lookup"=w2076, "Reads"=w2069, "ADCS Connection"=w2085, "Writes"=w2070) -> (w2057:T1)
        }
      }
      frame "StartRoutine" {
        n522 = in-place {
          in-place-border: w2146 -> [w2167]
          in-place-border: [w2160] -> w2145
          in-place-border: w2142 -> [w2165]
          w2148 = Type."Routine Start" ("Type")
          n523 = in-place-cluster #39(w2144) -> ("Status"=w2159:T26, "Parameters.Properties.Service Channels Status Lookup"=w2150:variant, "Service Channels Status"=w2149:T26, "Parameters.Properties.CAN.Diagnostic Protocol"=w2169:T6, "Parameters.Properties.Frames Lookup"=w2161:variant, "Reads"=w2156:T26, "ADCS Connection"=w2170:T19, "Writes"=w2154:T27)
          n524 = Unflatten From String(type=u16 0, binary string=w2165, error in (no error)=w2167) -> (value=w2151:u16, error out=w2155:errorcluster)  [unwired: 2 in, 1 out]
          n525 = call "Signals.Scale.Raw.vi"("Type"=w2148, "Lookup"=w2161, "error in"=w2155, "ID"=w2151, "Writes Ref"=w2154) -> ("error out"=w2164:errorcluster, "Data"=w2163:u8[])  [unwired: 5 in]
          n526 = case shown="\"UDS\"" w2169 {
            tunnel: [w2178 w2187 w2189] -> w2162
            tunnel: [w2177 w2185 w2188] -> w2168
            tunnel: w2164 -> [w2175 w2184 w2189]
            tunnel: w2170 -> [w2176 w2183 w2188]
            tunnel: [w2174 w2182 _] -> w2158
            tunnel: w2151 -> [w2173 w2181 _]
            tunnel: w2163 -> [w2172 w2180 _]
            tunnel: [w2171 w2179 _] -> w2157
            frame "KWP-2000" {
              n527 = call <vilib>:"StartRoutineByLocalIdentifier.vi"("error in (no error)"=w2175, "data in"=w2172, "local ID"=w2173, "diag ref in"=w2176) -> ("error out"=w2178:errorcluster, "success?"=w2174:bool, "data out"=w2171:u8[], "diag ref out"=w2177:T19)  [unwired: 4 in]
            }
            frame "UDS" {
              w2186 = u8 1 items=["Start routine"=1, "Stop routine"=2, "Request routine results"=3] ("mode")
              n528 = call <vilib>:"UDS RoutineControl.vi"("mode"=w2186, "error in (no error)"=w2184, "data in"=w2180, "ID"=w2181, "diag ref in"=w2183) -> ("error out"=w2187:errorcluster, "success?"=w2182:bool, "data out"=w2179:u8[], "diag ref out"=w2185:T19)  [unwired: 3 in]
            }
            frame "GMLAN", "User-Defined" {
            }
          }
          n529 = call "Signals.Scale.EU.vi"("Type"=w2148, "Lookup"=w2161, "error in (no error)"=w2162, "Unscaled Data"=w2157, "ID"=w2151, "Reads Ref"=w2156) -> ("error out"=w2153:errorcluster)  [unwired: 5 in]
          n530 = call "ServiceChannels.Status.Set.vi"("Type"=w2148, "Status Lookup"=w2150, "error in (no error)"=w2153, "ID"=w2151, "Service Channels Status Ref"=w2149) -> ("error out"=w2152:errorcluster)  [unwired: 6 in]
          n531 = in-place-cluster #39("Status"=w2159, "Parameters.Properties.Service Channels Status Lookup"=w2150, "Service Channels Status"=w2149, "Parameters.Properties.CAN.Diagnostic Protocol"=w2169, "Parameters.Properties.Frames Lookup"=w2161, "Reads"=w2156, "ADCS Connection"=w2168, "Writes"=w2154) -> (w2143:T1)
          n532 = call "Status.Set.vi"("error in (no error)"=w2152, "success?"=w2158, "Data"=w2157, "Status Ref"=w2159) -> ("error out"=w2160:errorcluster)  [unwired: 7 in]
        }
      }
      frame "RequestRoutineStatus" {
        n533 = in-place {
          in-place-border: w2194 -> [w2215]
          in-place-border: [w2207] -> w2192
          in-place-border: w2193 -> [w2213]
          w2196 = Type."Routine Request" ("Type")
          n534 = in-place-cluster #40(w2191) -> ("Status"=w2208:T26, "Parameters.Properties.Service Channels Status Lookup"=w2197:variant, "Service Channels Status"=w2198:T26, "Parameters.Properties.CAN.Diagnostic Protocol"=w2217:T6, "Parameters.Properties.Frames Lookup"=w2209:variant, "Reads"=w2202:T26, "ADCS Connection"=w2218:T19, "Writes"=w2203:T27)
          n535 = Unflatten From String(type=u16 0, binary string=w2213, error in (no error)=w2215) -> (value=w2199:u16, error out=w2204:errorcluster)  [unwired: 2 in, 1 out]
          n536 = call "Signals.Scale.Raw.vi"("Type"=w2196, "Lookup"=w2209, "error in"=w2204, "ID"=w2199, "Writes Ref"=w2203) -> ("error out"=w2212:errorcluster, "Data"=w2211:u8[])  [unwired: 5 in]
          n537 = case shown="\"KWP-2000\"" w2217 {
            tunnel: [w2222 w2234 w2236] -> w2210
            tunnel: [w2219 w2232 w2235] -> w2216
            tunnel: w2212 -> [w2224 w2231 w2236]
            tunnel: w2218 -> [w2223 w2230 w2235]
            tunnel: [w2221 w2229 _] -> w2206
            tunnel: w2199 -> [w2225 w2228 _]
            tunnel: w2211 -> [_ w2227 _]
            tunnel: [w2220 w2226 _] -> w2205
            frame "KWP-2000" {
              n538 = call <vilib>:"RequestRoutineResultsByLocalIdentifier.vi"("error in (no error)"=w2224, "local ID"=w2225, "diag ref in"=w2223) -> ("error out"=w2222:errorcluster, "success?"=w2221:bool, "data out"=w2220:u8[], "diag ref out"=w2219:T19)  [unwired: 5 in]
            }
            frame "UDS" {
              w2233 = u8 3 items=["Start routine"=1, "Stop routine"=2, "Request routine results"=3] ("mode")
              n539 = call <vilib>:"UDS RoutineControl.vi"("mode"=w2233, "error in (no error)"=w2231, "data in"=w2227, "ID"=w2228, "diag ref in"=w2230) -> ("error out"=w2234:errorcluster, "success?"=w2229:bool, "data out"=w2226:u8[], "diag ref out"=w2232:T19)  [unwired: 3 in]
            }
            frame "GMLAN", "User-Defined" {
            }
          }
          n540 = call "Signals.Scale.EU.vi"("Type"=w2196, "Lookup"=w2209, "error in (no error)"=w2210, "Unscaled Data"=w2205, "ID"=w2199, "Reads Ref"=w2202) -> ("error out"=w2201:errorcluster)  [unwired: 5 in]
          n541 = call "ServiceChannels.Status.Set.vi"("Type"=w2196, "Status Lookup"=w2197, "error in (no error)"=w2201, "ID"=w2199, "Service Channels Status Ref"=w2198) -> ("error out"=w2200:errorcluster)  [unwired: 6 in]
          n542 = call "Status.Set.vi"("error in (no error)"=w2200, "success?"=w2206, "Data"=w2205, "Status Ref"=w2208) -> ("error out"=w2207:errorcluster)  [unwired: 7 in]
          n543 = in-place-cluster #40("Status"=w2208, "Parameters.Properties.Service Channels Status Lookup"=w2197, "Service Channels Status"=w2198, "Parameters.Properties.CAN.Diagnostic Protocol"=w2217, "Parameters.Properties.Frames Lookup"=w2209, "Reads"=w2202, "ADCS Connection"=w2216, "Writes"=w2203) -> (w2190:T1)
        }
      }
      frame "StopRoutine" {
        n544 = in-place {
          in-place-border: w2240 -> [w2262]
          in-place-border: [w2255] -> w2237
          in-place-border: w2239 -> [w2260]
          w2243 = Type."Routine Stop" ("Type")
          n545 = in-place-cluster #41(w2241) -> ("Status"=w2254:T26, "Parameters.Properties.Service Channels Status Lookup"=w2244:variant, "Service Channels Status"=w2245:T26, "Parameters.Properties.CAN.Diagnostic Protocol"=w2264:T6, "Parameters.Properties.Frames Lookup"=w2256:variant, "Reads"=w2249:T26, "ADCS Connection"=w2265:T19, "Writes"=w2250:T27)
          n546 = Unflatten From String(type=u16 0, binary string=w2260, error in (no error)=w2262) -> (value=w2246:u16, error out=w2251:errorcluster)  [unwired: 2 in, 1 out]
          n547 = call "Signals.Scale.Raw.vi"("Type"=w2243, "Lookup"=w2256, "error in"=w2251, "ID"=w2246, "Writes Ref"=w2250) -> ("error out"=w2259:errorcluster, "Data"=w2258:u8[])  [unwired: 5 in]
          n548 = case shown="\"KWP-2000\"" w2264 {
            tunnel: [w2269 w2282 w2284] -> w2257
            tunnel: [w2272 w2280 w2283] -> w2263
            tunnel: w2259 -> [w2268 w2279 w2284]
            tunnel: w2265 -> [w2273 w2278 w2283]
            tunnel: [w2270 w2277 _] -> w2253
            tunnel: w2246 -> [w2267 w2276 _]
            tunnel: w2258 -> [w2266 w2275 _]
            tunnel: [w2271 w2274 _] -> w2252
            frame "KWP-2000" {
              n549 = call <vilib>:"StopRoutineByLocalIdentifier.vi"("error in (no error)"=w2268, "data in"=w2266, "local ID"=w2267, "diag ref in"=w2273) -> ("error out"=w2269:errorcluster, "success?"=w2270:bool, "data out"=w2271:u8[], "diag ref out"=w2272:T19)  [unwired: 4 in]
            }
            frame "UDS" {
              w2281 = u8 2 items=["Start routine"=1, "Stop routine"=2, "Request routine results"=3] ("mode")
              n550 = call <vilib>:"UDS RoutineControl.vi"("mode"=w2281, "error in (no error)"=w2279, "data in"=w2275, "ID"=w2276, "diag ref in"=w2278) -> ("error out"=w2282:errorcluster, "success?"=w2277:bool, "data out"=w2274:u8[], "diag ref out"=w2280:T19)  [unwired: 3 in]
            }
            frame "GMLAN", "User-Defined" {
            }
          }
          n551 = call "Signals.Scale.EU.vi"("Type"=w2243, "Lookup"=w2256, "error in (no error)"=w2257, "Unscaled Data"=w2252, "ID"=w2246, "Reads Ref"=w2249) -> ("error out"=w2248:errorcluster)  [unwired: 5 in]
          n552 = call "ServiceChannels.Status.Set.vi"("Type"=w2243, "Status Lookup"=w2244, "error in (no error)"=w2248, "ID"=w2246, "Service Channels Status Ref"=w2245) -> ("error out"=w2247:errorcluster)  [unwired: 6 in]
          n553 = call "Status.Set.vi"("error in (no error)"=w2247, "success?"=w2253, "Data"=w2252, "Status Ref"=w2254) -> ("error out"=w2255:errorcluster)  [unwired: 7 in]
          n554 = in-place-cluster #41("Status"=w2254, "Parameters.Properties.Service Channels Status Lookup"=w2244, "Service Channels Status"=w2245, "Parameters.Properties.CAN.Diagnostic Protocol"=w2264, "Parameters.Properties.Frames Lookup"=w2256, "Reads"=w2249, "ADCS Connection"=w2263, "Writes"=w2250) -> (w2238:T1)
        }
      }
    }
    n555 = disable-structure shown="DebugRT==TRUE" {
      disable-tunnel: w66 -> [w72 w77]
      disable-tunnel: [w72 w77] -> w59
      frame condition #0 {
        n556 = case shown="Default" w72 {
          selector: w72 -> [_ w74]
          frame "" {
          }
          frame Default {
            n557 = Concatenate Strings(w74, "Started" ("string"), "\r\n") -> (w76:string)
            n558 = call <vilib>:"NI VeriStand - Print Debug String.vi"("Message"=w76) -> ()  [unwired: 10 in, 1 out]
          }
        }
      }
      frame condition #1 (active) {
      }
    }
    n559 = Unbundle By Name(w56) -> ("TesterPresentEnabled?"=w55:bool)
    n560 = call "ADCS.TesterPresent.vi"("Enabled?"=w55, "error in (no error)"=w58, "Reset"=w57, "State Variables in"=w62) -> ("error out"=w50:errorcluster, "State Variables out"=w61:T1)  [unwired: 6 in]
    n561 = call "Restart.LocalStop.Read.vi"("error in (no error)"=w50, "Data Value Reference in"=w45) -> ("error out"=w49:errorcluster, "LocalStop"=w47:bool)  [unwired: 8 in]
    n562 = call <vilib>:"Async.Processes.Report.vi"("Error"=w49, "Stop Async on Error?"=FALSE ("Stop on Error?"), "Process in"=w54) -> ("Stop"=w48:bool)  [unwired: 7 in, 1 out]
    n563 = disable-structure shown="DebugRT==TRUE" {
      disable-tunnel: w59 -> [w78 _]
      disable-tunnel: w49 -> [_ _]
      frame condition #0 {
        n564 = case shown="Default" w78 {
          selector: w78 -> [_ w80]
          frame "" {
          }
          frame Default {
            n565 = Concatenate Strings(w80, "Finished" ("string"), "\r\n") -> (w82:string)
            n566 = call <vilib>:"NI VeriStand - Print Debug String.vi"("Message"=w82) -> ()  [unwired: 10 in, 1 out]
          }
        }
      }
      frame condition #1 (active) {
      }
    }
    n567 = Compound Arithmetic op=OR(w47, w48) -> (w46:bool)
  }
  "error out" <- w29
